vi "运维调试_五参数.vi"() -> ()   [LabVIEW 2016, in "斯坦道多参数.lvlib"]
uses:
  <vilib>/Utility/miscctls.llb/LVPointTypeDef.ctl
  <vilib>/Utility/config.llb/NI_LVConfig.lvlib
panel:
  out "串口号":string
  in  "水深写入":bool
  in  "水深读取":bool
  in  "水深校准":dbl caption="水深校准:"
  in  "仪器参数设置":bool
  out "模块版本号":string
  in  "写入":bool
  in  "读取":bool
  in  "B":dbl caption="校准值B:"
  in  "K":dbl caption="校准值K:"
  in  "标样核查":bool
  in  "串口设置":bool
  in  "质控参数设置":bool
  in  "打开串口":bool
  in  "释放串口":bool
  out "多参数横条运行状态":T1(xcontrol)
  in  "数据区":i32(listbox)
  in  "停止测量(单探)":bool
  in  "启动测量(单探)":bool
  in  "控制命令区探头选择":u16(ring)=9 items=["氨氮"=3, "水温"=9, "pH值"=10, "溶解氧"=11, "电导率"=12, "浊度"=13, "叶绿素a"=14, "藻密度"=15, "蓝绿藻"=16, "氧化还原电位"=17, "溶解氧%"=18, "盐度"=19]
  in  "同步时间":bool
  in  "初始化(清洗)":bool
  in  "停止测量(全部)":bool
  in  "启动测量(全部)":bool
  in  "关键参数区读取":bool
  in  "关键参数区":i32(listbox)
  in  "传感器参数读取":bool
  in  "传感器区":i32(listbox)
  in  "返回":bool
  in  "设置":bool
  out "运行状态":string
  in  "停止":bool
  in  "水样测试":bool
  out "集成报警信息":string
  # "控制命令区"
  # "探头校准"
  # "水深校准"
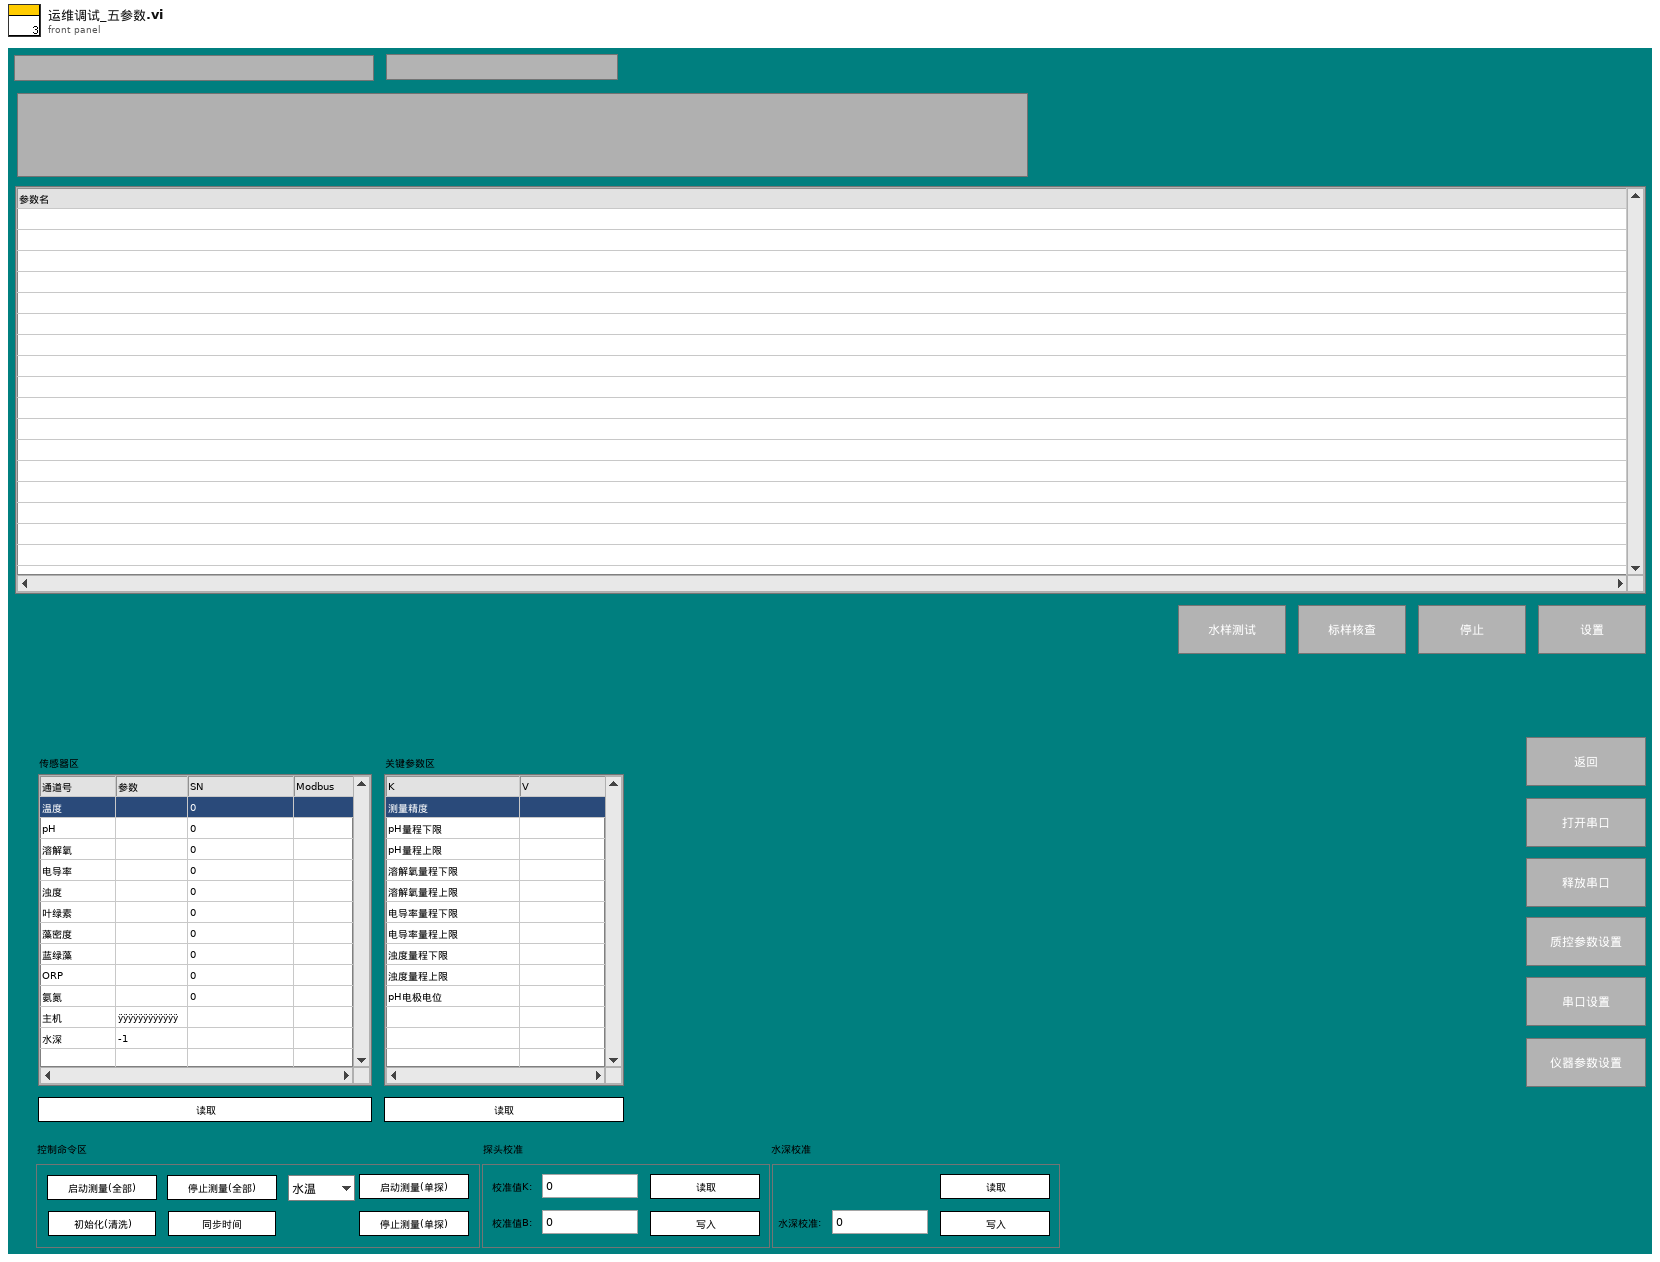
[diagram p1: front panel]
types:
  T1 = cluster{"系统时间":timestamp, "工作状态":u16, "测量模式":u16, "告警代码":enum16{"无告警", "缺试剂告警", "缺水样告警", "缺蒸馏水告警", "缺标液告警", "仪表漏液告警", "标定异常告警", "超量程告警", "加热异常", "低试剂预警", "超上限告警", "超下限告警", "仪表内部其他异常", "滴定异常告警", "电极异常告警", "量程切换告警", "参数设置告警", "PH电极电位异常", "电导率电极异常", "浊度光度异常", "溶解氧电极异常", "溶解氧光强异常", "温度异常告警", "PH异常告警", "溶解氧异常告警", "电导率异常告警", "浊度异常告警", "叶绿素异常告警", "藻密度异常告警", "蓝绿藻异常告警", "ORP异常告警", "氨氮异常告警", "清洁刷异常告警", "SD卡异常告警", "蓝牙异常告警", "Wifi异常告警", "流程异常告警"}, "故障代码":enum16{"无故障", "电机故障", "温度故障", "通讯故障", "滴定故障"}, "日志代码":u16, "软件版本":string}
  T2 = typedef "斯坦道多参数.lvlib/水样测试启动自定义输入参数.ctl" = cluster{"测量模式":enum16{"待机", "水样测试", "标样核查", "零点核查", "跨度核查", "空白测试", "平行样测试", "加标回收", "空白校准", "标样校准", "初始化（清洗）"}, "数据类型":string, "手动启动标记":bool, "测量时间":dbl}
  T3 = typedef "LVPointTypeDef.ctl" = cluster{"Horizontal":i16, "Vertical":i16}
  T4 = cluster{"时间标识":timestamp, "设备":string, "日志信息":string}
  T5 = enum16{"无告警", "缺试剂告警", "缺水样告警", "缺蒸馏水告警", "缺标液告警", "仪表漏液告警", "标定异常告警", "超量程告警", "加热异常", "低试剂预警", "超上限告警", "超下限告警", "仪表内部其他异常", "滴定异常告警", "电极异常告警", "量程切换告警", "参数设置告警", "PH电极电位异常", "电导率电极异常", "浊度光度异常", "溶解氧电极异常", "溶解氧光强异常", "温度异常告警", "PH异常告警", "溶解氧异常告警", "电导率异常告警", "浊度异常告警", "叶绿素异常告警", "藻密度异常告警", "蓝绿藻异常告警", "ORP异常告警", "氨氮异常告警", "清洁刷异常告警", "SD卡异常告警", "蓝牙异常告警", "Wifi异常告警", "流程异常告警"}
  T6 = cluster{"水温":dbl, "pH":dbl, "DO":dbl, "Cond":dbl, "Turb":dbl, "叶绿素":dbl, "藻密度":dbl, "蓝绿藻":dbl, "ORP":dbl, "NH3N":dbl}
  T7 = cluster{"因子编码":string, "单位":string, "标样参考值":sgl, "水样数据时间":timestamp, "水样实测值":sgl, "水样数据标识":string, "K":sgl, "B":sgl, "T":sgl, "H":sgl, "水深":sgl, "探头温度":sgl}
  T8 = typedef "NI_LVConfig.lvlib/Config Data RefNum.ctl" = refnum<k1>
  T9 = cluster{"测量量程":dbl, "测量精度":dbl, "测量间隔":dbl, "消解温度":dbl, "消解时长":dbl, "空白校准时间":timestamp, "曲线截距":dbl, "曲线斜率":dbl, "测量检出限":dbl, "测量信号值":dbl, "线性相关系数":dbl, "二次多项式系数":dbl, "标样校准时间":timestamp, "稀释倍数":dbl, "三项式系数":dbl, "空白标定系数":dbl, "量程系数":dbl, "F0/ORPA":dbl, "F1/ORPB":dbl, "F2/ORPK":dbl, "F3":dbl, "F4":dbl, "F5":dbl, "F6":dbl, "F7":dbl, "X0/滴定数":dbl, "量程":dbl}
  T10 = cluster{"测量量程":dbl, "测量精度":dbl, "测量间隔":dbl, "消解温度":dbl, "消解时长":dbl, "空白校准时间":timestamp, "曲线截距":dbl, "曲线斜率":dbl, "测量检出限":dbl, "测量信号值":dbl, "线性相关系数":dbl, "二次多项式系数":dbl, "标样校准时间":timestamp, "稀释倍数":dbl, "三项式系数":dbl, "空白标定系数":dbl, "量程系数":dbl, "F0/ORPA":dbl, "F1/ORPB":dbl, "F2/ORPK":dbl, "F3":dbl, "F4":dbl, "F5":dbl, "F6":dbl, "F7":dbl, "X0/滴定数":dbl, "量程":dbl}[]
  T11 = cluster{"因子编码":string, "单位":string, "标样参考值":sgl, "水样数据时间":timestamp, "水样实测值":sgl, "水样数据标识":string, "K":sgl, "B":sgl, "T":sgl, "H":sgl, "水深":sgl, "探头温度":sgl}[]
  T12 = enum8{"Enabled", "Disabled", "Disabled and Grayed Out"}
  T13 = typedef "斯坦道多参数.lvlib/标样核查启动自定义输入参数.ctl" = cluster{"测量模式":enum16{"待机", "水样测试", "标样核查", "零点核查", "跨度核查", "空白测试", "平行样测试", "加标回收", "空白校准", "标样校准", "初始化（清洗）"}, "数据标记表":string, "输出参数":cluster{"水温":bool, "pH":bool, "DO":bool, "浊度":bool, "电导率":bool, "保存组数":dbl}}
  T14 = cluster{"水温标准液标准浓度":dbl, "酸碱度标准液标准浓度":dbl, "溶解氧标准液标准浓度":dbl, "电导率标准液标准浓度":dbl, "浊度标准液标准浓度":dbl}
  T15 = cluster{"确定":bool, "水温标准液标准浓度":dbl, "酸碱度标准液标准浓度":dbl, "溶解氧标准液标准浓度":dbl, "电导率标准液标准浓度":dbl, "浊度标准液标准浓度":dbl}
  T16 = cluster{"运行模式":enum16{"维护模式", "常规模式", "应急模式", "质控模式"}, "24H周期设置":bool[]}
  T17 = cluster{"水温":bool, "pH":bool, "DO":bool, "浊度":bool, "电导率":bool, "保存组数":dbl}
  T18 = enum32{"Bad", "Idle", "Run top level", "Running"}
  T19 = cluster{"Major":u16, "Minor":u16, "Fix":u16, "Build":u16}
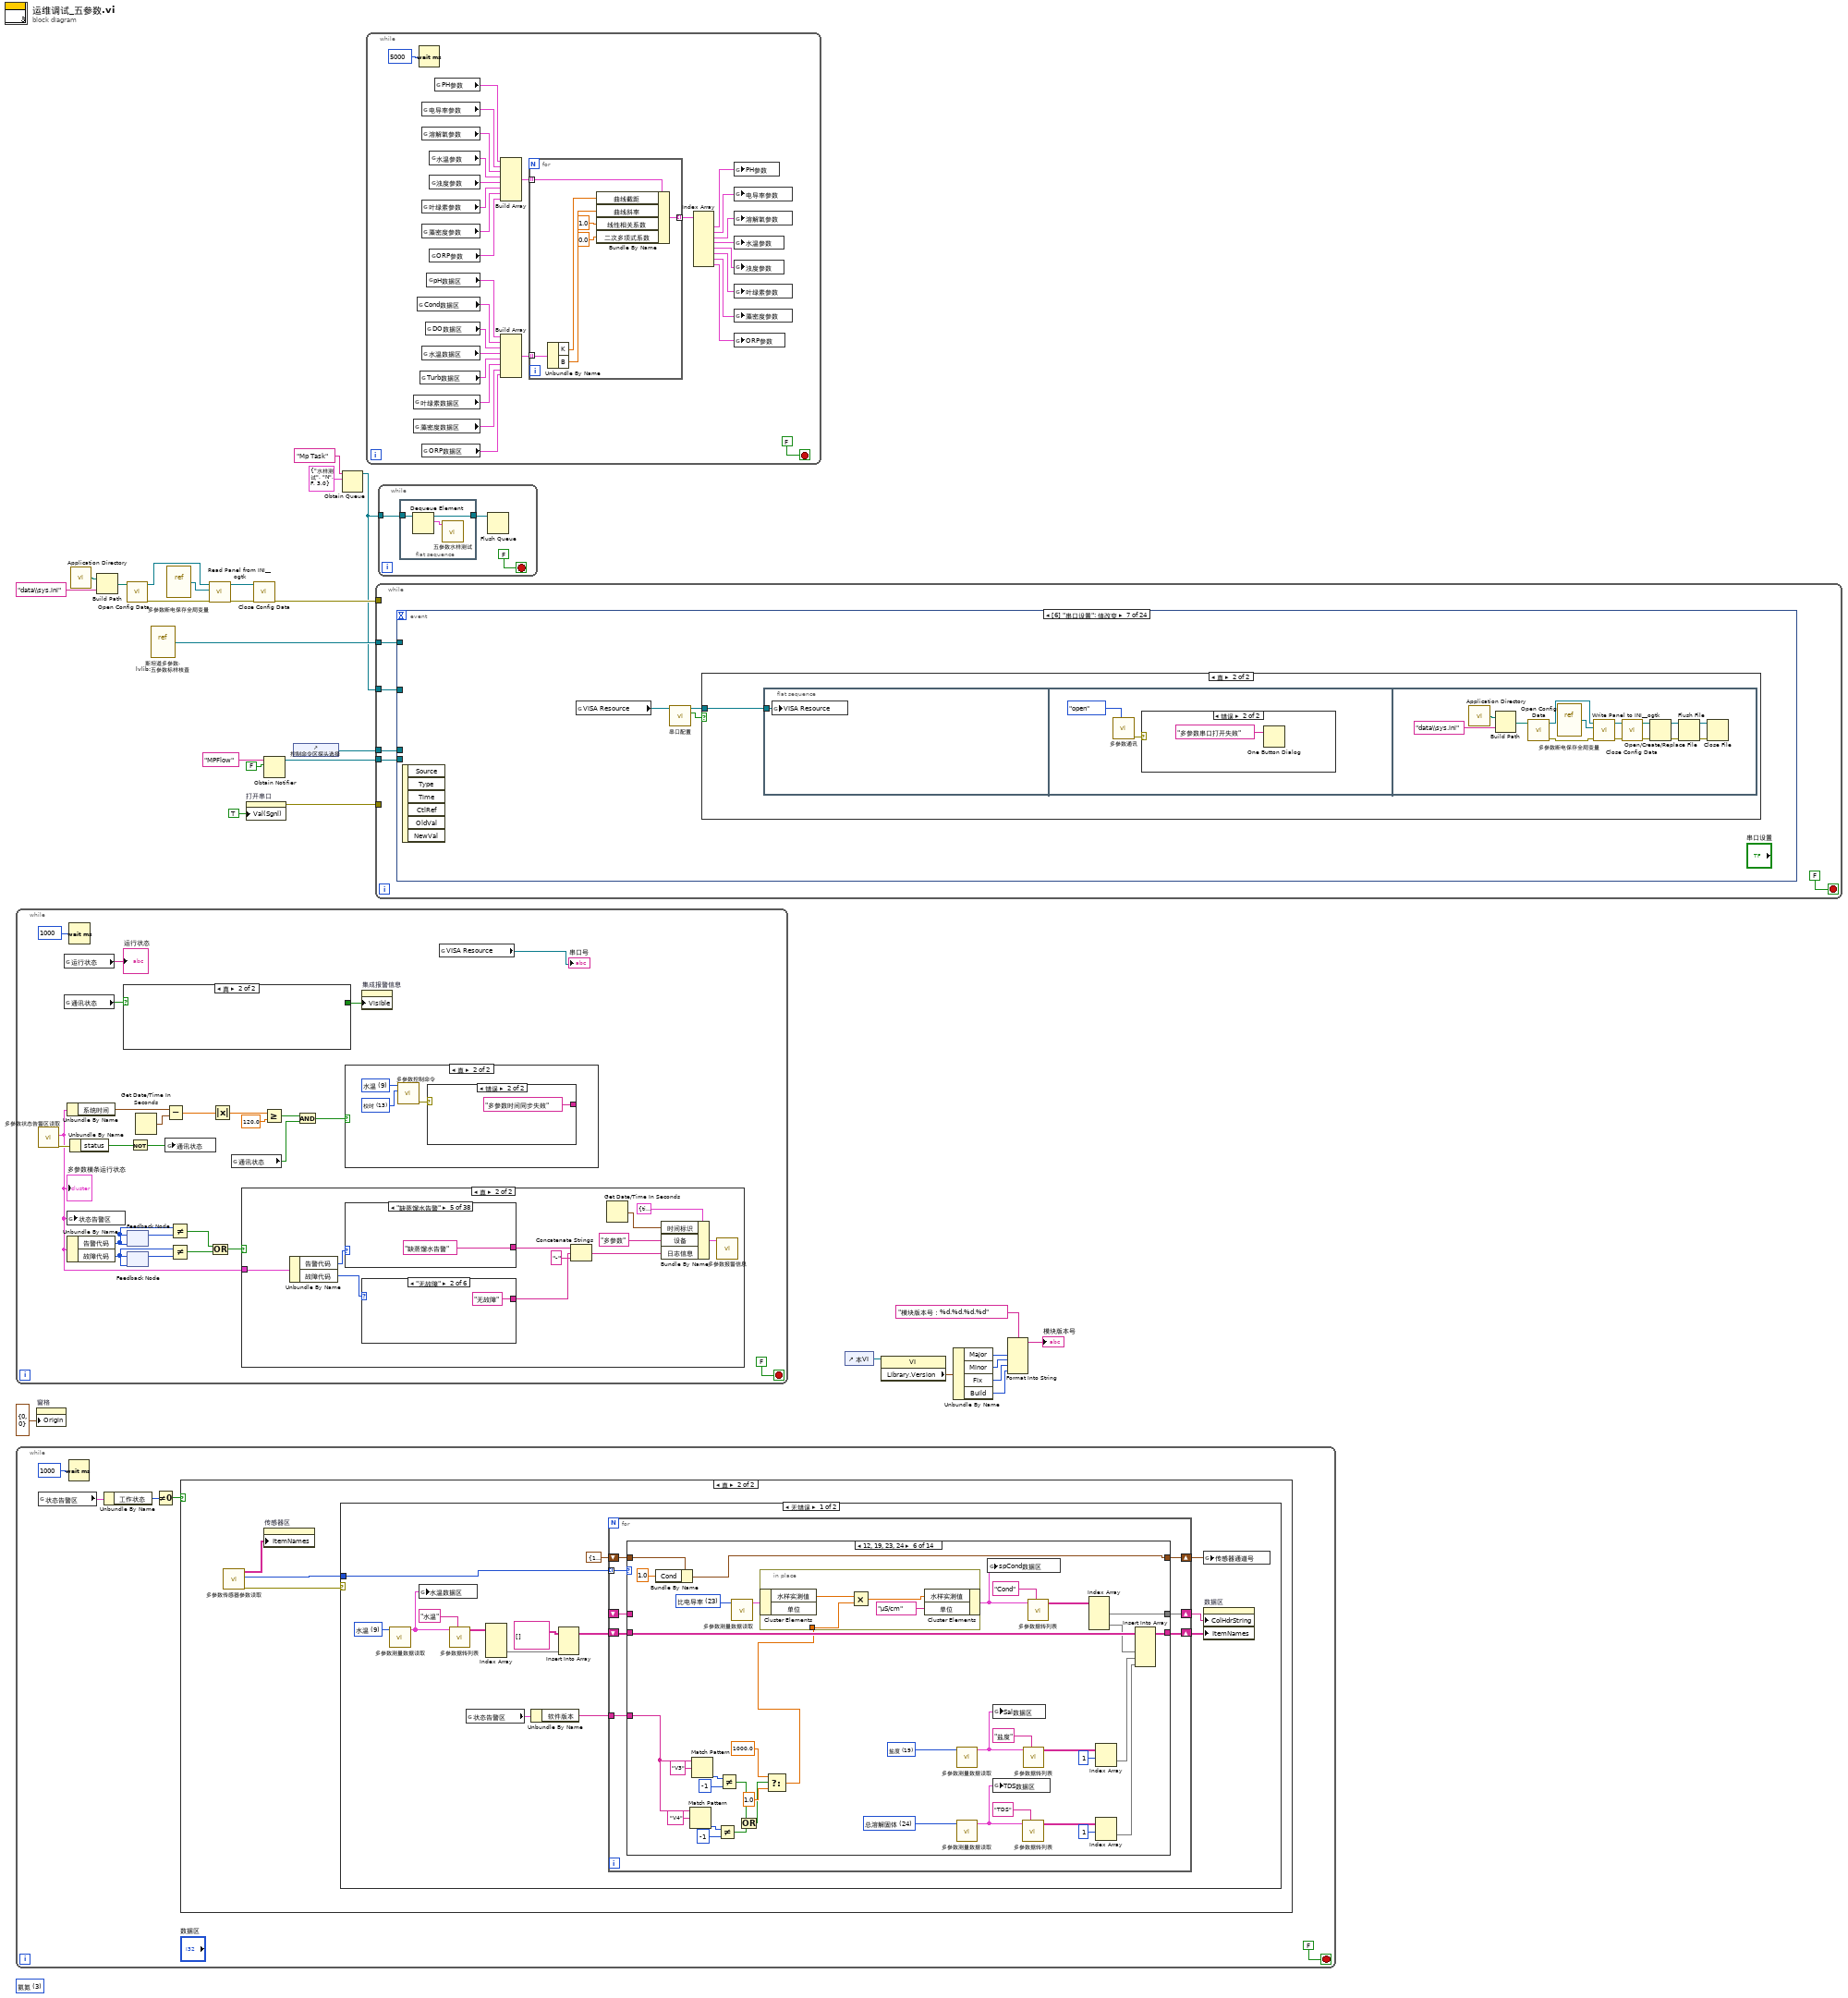
[diagram p0: block diagram]
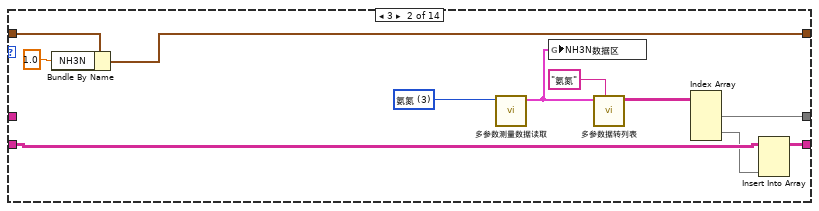
[diagram p4: hidden frame]
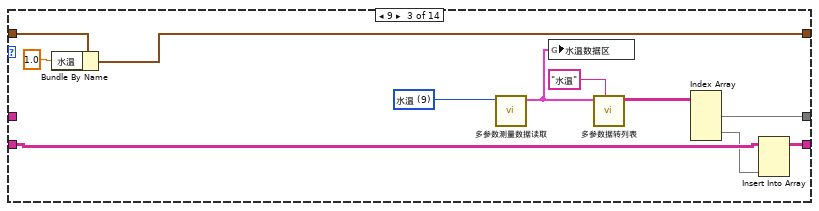
[diagram p5: hidden frame]
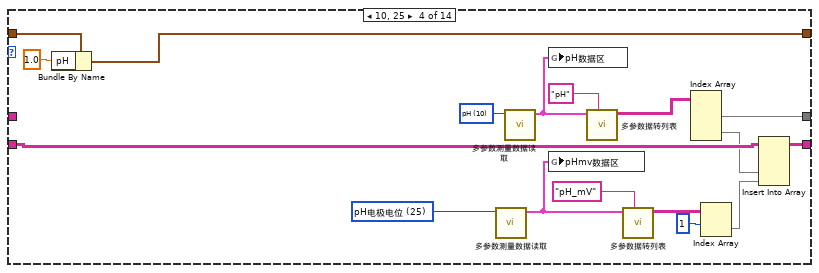
[diagram p6: hidden frame]
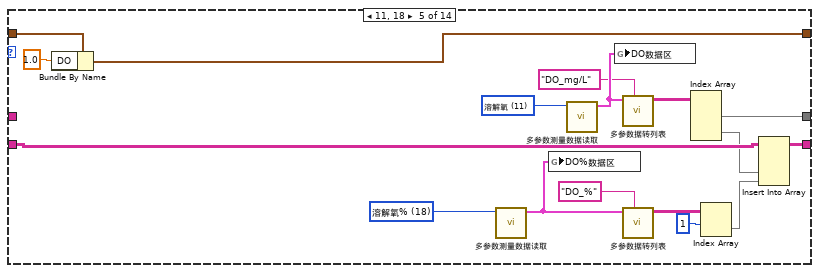
[diagram p7: hidden frame]
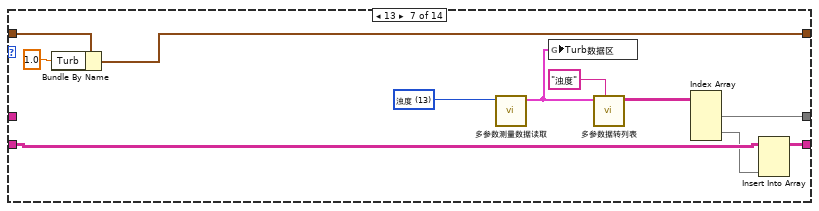
[diagram p8: hidden frame]
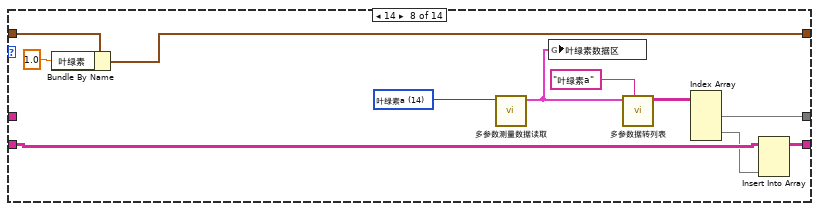
[diagram p9: hidden frame]
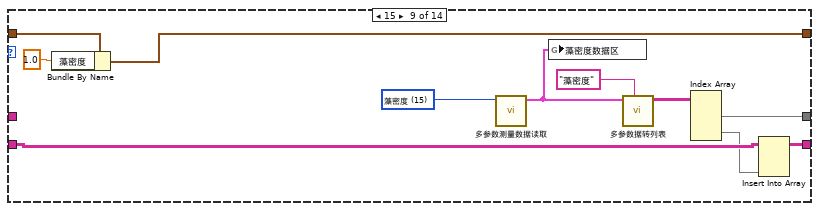
[diagram p10: hidden frame]
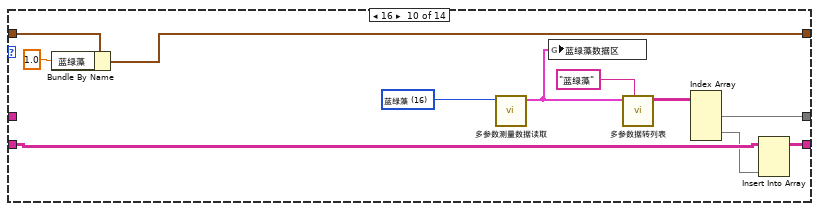
[diagram p11: hidden frame]
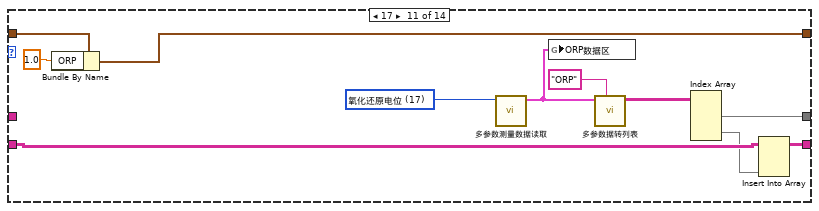
[diagram p12: hidden frame]
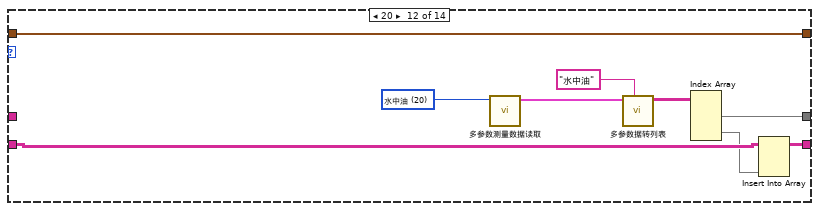
[diagram p13: hidden frame]
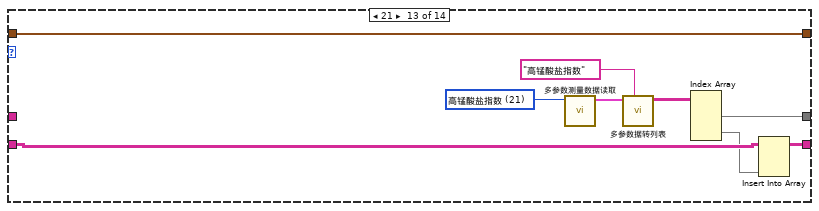
[diagram p14: hidden frame]
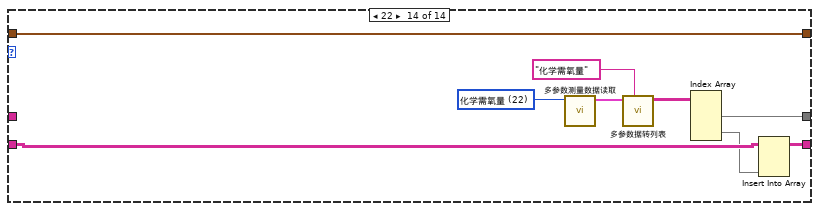
[diagram p15: hidden frame]
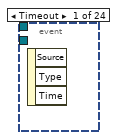
[diagram p17: hidden frame]
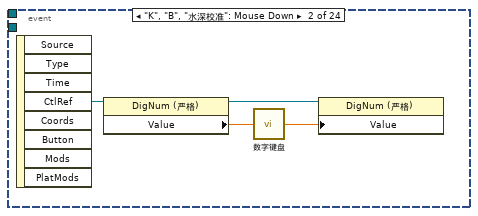
[diagram p18: hidden frame]
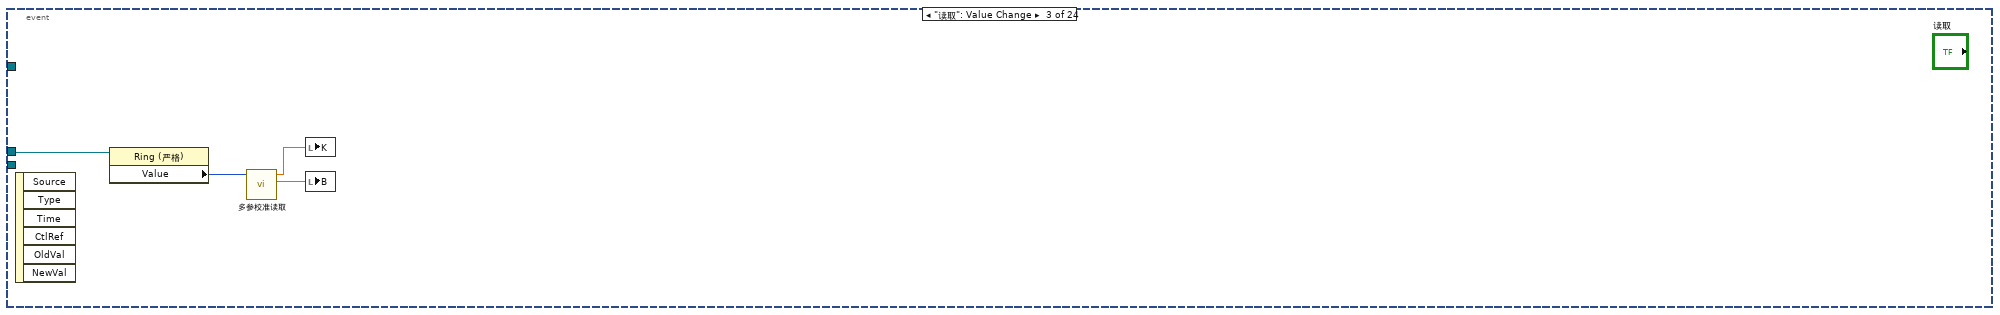
[diagram p19: hidden frame]
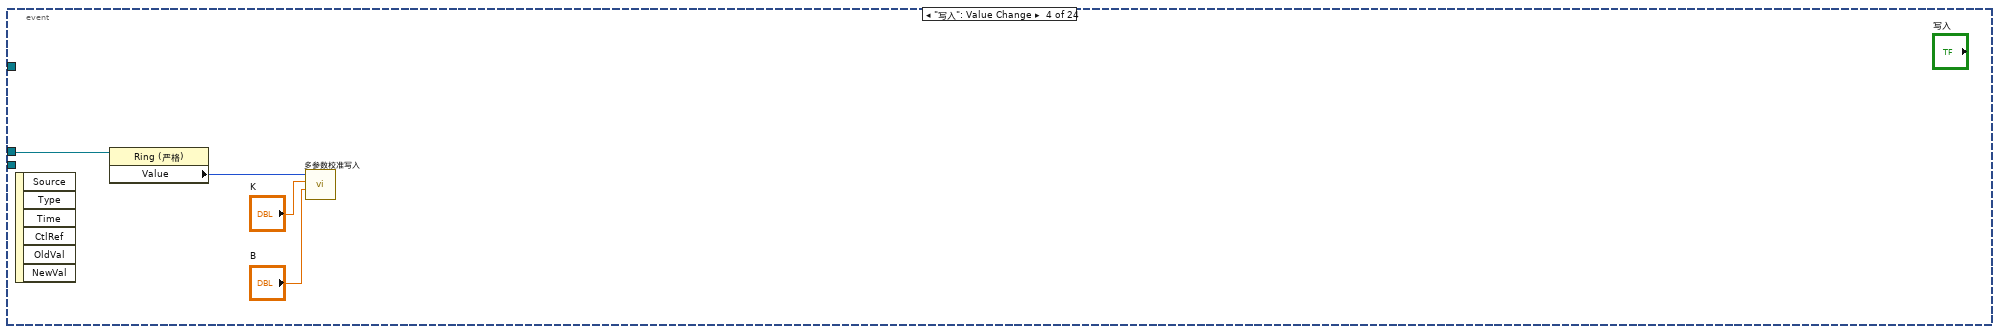
[diagram p20: hidden frame]
diagram:
  (unwired) u16 3 items=["氨氮"=3, "水温"=9, "pH"=10, "溶解氧"=11, "电导率"=12, "浊度"=13, "叶绿素a"=14, "藻密度"=15, "蓝绿藻"=16, "氧化还原电位"=17, "溶解氧%"=18, "盐度"=19, "水中油"=20, "高锰酸盐指数"=21, "化学需氧量"=22, "比电导率"=23, "总溶解固体"=24, "pH电极电位"=25] ("下拉列表")
  n1 = while {
    stop <- FALSE stop-if-true
    n2 = call "多参数状态告警区读取.vi"() -> ("error out"=w41:errorcluster, "状态告警块"=w38:T1)  [unwired: 9 in, 1 out]
    "多参数横条运行状态" <- w38
    n3 = global read "多参数全局变量.vi" "运行状态"() -> (→"运行状态":string)
    n4 = global read "多参数全局变量.vi" "通讯状态"() -> (w51:bool)
    n5 = Unbundle By Name(w38) -> ("系统时间"=w37:timestamp)
    n6 = global write "多参数全局变量.vi" "状态告警区"(w38) -> ()
    n7 = Unbundle By Name(w38) -> ("告警代码"=w47:T5, "故障代码"=w45:enum16{"无故障", "电机故障", "温度故障", "通讯故障", "滴定故障"})
    n8 = Wait (ms)(milliseconds to wait=u32 1000 ("等待时间（毫秒）")) -> ()  [unwired: 1 out]
    n9 = Unbundle By Name(w41) -> ("status"=w40:bool)
    n10 = case shown="真" w51 {
      tunnel: [TRUE ("可见") _] -> w50
      frame False {
        "集成报警信息" <- "通讯异常" ("集成报警信息")
      }
      frame True {
      }
    }
    n11 = feedback #1(w47) -> (w48:T5)
    n12 = feedback-in #1(w47) -> ()
    n13 = feedback #2(w45) -> (w46:enum16{"无故障", "电机故障", "温度故障", "通讯故障", "滴定故障"})
    n14 = feedback-in #2(w45) -> ()
    n15 = Not(x=w40) -> (.not. x?=w39:bool)
    n16 = Get Date/Time In Seconds() -> (seconds since 1Jan1904=w36:timestamp)
    n17 = Subtract(x=w37, y=w36) -> (x-y=w35:dbl)
    n18 = global write "多参数全局变量.vi" "通讯状态"(w39) -> ()
    n19 = Not Equal?(x=w47, y=w48) -> (x != y?=w43:bool)
    n20 = Not Equal?(x=w45, y=w46) -> (x != y?=w44:bool)
    n21 = Or(x=w43, y=w44) -> (x .or. y?=w42:bool)
    n22 = Absolute Value(x=w35) -> (abs(x)=w34:dbl)
    n23 = global read "多参数全局变量.vi" "通讯状态"() -> (w30:bool)
    n24 = case shown="真" w42 {
      tunnel: w38 -> [_ w69]
      frame False {
      }
      frame True {
        n25 = Unbundle By Name(w69) -> ("告警代码"=w68:T5, "故障代码"=w67:enum16{"无故障", "电机故障", "温度故障", "通讯故障", "滴定故障"})
        n26 = case shown="\"缺蒸馏水告警\"" w68 {
          selector: w68 -> [w80 _ _ _ _ _ _ _ _ _ _ _ _ _ _ _ _ _ _ _ _ _ _ _ _ _ _ _ _ _ _ _ _ _ _ _ _ _]
          tunnel: [w79 "无告警" "缺试剂告警" "缺水样告警" "缺蒸馏水告警" "缺标液告警" "仪表漏液告警" "标定异常告警" "超量程告警" "加热异常" "低试剂预警" "超上限告警" "超下限告警" "仪表内部其他异常" "滴定异常告警" "电极异常告警" "量程切换告警" "参数设置告警" "PH电极电位异常" "电导率电极异常" "浊度光度异常" "溶解氧电极异常" "溶解氧光强异常" "温度异常告警" "PH异常告警" "溶解氧异常告警" "电导率异常告警" "浊度异常告警" "叶绿素异常告警" "藻密度异常告警" "蓝绿藻异常告警" "ORP异常告警" "氨氮异常告警" "清洁刷异常告警" "SD卡异常告警" "蓝牙异常告警" "WiFi异常告警" "流程异常告警"] -> w66
          frame Default {
            n27 = Format Into String(format string="%d" ("格式字符串"), initial string="未知" ("工作状态"), w80) -> (resulting string=w79:string)  [unwired: 1 in, 1 out]
          }
          frame "无告警" {
          }
          frame "缺试剂告警" {
          }
          frame "缺水样告警" {
          }
          frame "缺蒸馏水告警" {
          }
          frame "缺标液告警" {
          }
          frame "仪表漏液告警" {
          }
          frame "标定异常告警" {
          }
          frame "超量程告警" {
          }
          frame "加热异常" {
          }
          frame "低试剂预警" {
          }
          frame "超上限告警" {
          }
          frame "超下限告警" {
          }
          frame "仪表内部其他异常" {
          }
          frame "滴定异常告警" {
          }
          frame "电极异常告警" {
          }
          frame "量程切换告警" {
          }
          frame "参数设置告警" {
          }
          frame "PH电极电位异常" {
          }
          frame "电导率电极异常" {
          }
          frame "浊度光度异常" {
          }
          frame "溶解氧电极异常" {
          }
          frame "溶解氧光强异常" {
          }
          frame "温度异常告警" {
          }
          frame "PH异常告警" {
          }
          frame "溶解氧异常告警" {
          }
          frame "电导率异常告警" {
          }
          frame "浊度异常告警" {
          }
          frame "叶绿素异常告警" {
          }
          frame "藻密度异常告警" {
          }
          frame "蓝绿藻异常告警" {
          }
          frame "ORP异常告警" {
          }
          frame "氨氮异常告警" {
          }
          frame "清洁刷异常告警" {
          }
          frame "SD卡异常告警" {
          }
          frame "蓝牙异常告警" {
          }
          frame "Wifi异常告警" {
          }
          frame "流程异常告警" {
          }
        }
        n28 = case shown="\"无故障\"" w67 {
          selector: w67 -> [w71 _ _ _ _ _]
          tunnel: [w70 "无故障" "电机故障" "温度故障" "通讯故障" "滴定故障"] -> w65
          frame Default {
            n29 = Format Into String(format string="%d" ("格式字符串"), initial string="未知" ("工作状态"), w71) -> (resulting string=w70:string)  [unwired: 1 in, 1 out]
          }
          frame "无故障" {
          }
          frame "电机故障" {
          }
          frame "温度故障" {
          }
          frame "通讯故障" {
          }
          frame "滴定故障" {
          }
        }
        n30 = Concatenate Strings(w66, "-" ("字符串"), w65) -> (w61:string)
        n31 = Get Date/Time In Seconds() -> (seconds since 1Jan1904=w60:timestamp)
        n32 = Bundle By Name(cluster=T4 {"时间标识"=timestamp(0 s since 1904-01-01), "设备"="", "日志信息"=""} ("data in"), "时间标识"=w60, "设备"="多参数", "日志信息"=w61) -> (w62:T4)
        n33 = call "多参数报警信息.vi"("data in"=w62) -> ()  [unwired: 10 in, 1 out]
      }
    }
    n34 = Greater Or Equal?(x=w34, y=120.0) -> (x >= y?=w33:bool)
    n35 = And(x=w33, y=w30) -> (x .and. y?=w31:bool)
    n36 = case shown="真" w31 {
      frame False {
      }
      frame True {
        w54 = u16 13 items=["启动测量（全部）"=1, "初始化（清洗）"=10, "停止测量（全部）"=11, "校时"=13, "启动测量（单个传感器）"=19, "停止测量（单个传感器）"=20] ("控制命令")
        w55 = u16 9 items=["氨氮"=3, "水温"=9, "pH值"=10, "溶解氧"=11, "电导率"=12, "浊度"=13, "叶绿素a"=14, "藻密度"=15, "蓝绿藻"=16, "氧化还原电位"=17, "溶解氧%"=18, "盐度"=19] ("站号")
        n37 = call "多参数控制命令.vi"("控制命令"=w54, "站号"=w55) -> ("error out"=w56:errorcluster)  [unwired: 9 in]
        n38 = case shown="错误" w56 {
          tunnel: ["多参数时间同步成功" ("消息") "多参数时间同步失败" ("消息")] -> _
          frame No Error {
          }
          frame Error {
          }
        }
      }
    }
    n39 = property on="集成报警信息" class="Str"("Visible"=w50) -> ()  [unwired: 2 in, 2 out]
    n40 = global read "多参数断电保存全局变量.vi" "VISA Resource"() -> (→"串口号":refnum<visa-resource-name>)
  }
  n41 = while {
    stop <- FALSE stop-if-true
    n42 = global read "多参数全局变量.vi" "状态告警区"() -> (w124:T1)
    n43 = Wait (ms)(milliseconds to wait=u32 1000 ("等待时间（毫秒）")) -> ()  [unwired: 1 out]
    n44 = Unbundle By Name(w124) -> ("工作状态"=w123:u16)
    n45 = Not Equal To 0?(x=w123) -> (x != 0?=w122:bool)
    n46 = case shown="真" w122 {
      frame False {
      }
      frame True {
        n47 = call "多参数传感器参数读取.vi"() -> ("error out"=w129:errorcluster, "modbus"=w128:u16[], "添加的数组"=w127:string[][])  [unwired: 9 in]
        n48 = property on="传感器区" class="MCListbox (严格)"("ItemNames"=w127) -> ()  [unwired: 2 in, 2 out]
        n49 = case shown="无错误" w129 {
          tunnel: w128 -> [w143 _]
          frame No Error {
            w140 = u16 9 items=["氨氮"=3, "水温"=9, "pH"=10, "溶解氧"=11, "电导率"=12, "浊度"=13, "叶绿素a"=14, "藻密度"=15, "蓝绿藻"=16, "氧化还原电位"=17, "溶解氧%"=18, "盐度"=19, "水中油"=20, "高锰酸盐指数"=21, "化学需氧量"=22, "比电导率"=23, "总溶解固体"=24, "pH电极电位"=25] ("下拉列表")
            n50 = call "多参数测量数据读取.vi"("探头选择"=w140) -> ("测量数据块"=w135:T7)  [unwired: 8 in, 2 out]
            n51 = global write "多参数全局变量.vi" "水温数据区"(w135) -> ()
            n52 = call "多参数据转列表.vi"("参数名"="水温", "测量数据块"=w135) -> ("添加的数组"=w133:string[][])  [unwired: 9 in]
            n53 = global read "多参数全局变量.vi" "状态告警区"() -> (w131:T1)
            n54 = Index Array(array=w133) -> (element #2=w132:string[])  [unwired: 4 in, 1 out]
            n55 = Unbundle By Name(w131) -> ("软件版本"=w130:string)
            n56 = Insert Into Array(array=string[][] [] ("子数组"), new element=w132) -> (w138:string[][])  [unwired: 2 in]
            n57 = for {
              tunnel: w143 -> [w151] mode=indexing
              shift-right: [w149] -> w141
              shift-left: w138 -> [w150]
              shift-right: [w148] -> w142
              shift-left: _ -> [w147]
              shift-right: [w146] -> w136
              shift-left: T6 {"水温"=1.0, "pH"=0.0, "DO"=0.0, "Cond"=0.0, "Turb"=0.0, "叶绿素"=0.0, "藻密度"=0.0, "蓝绿藻"=0.0, "ORP"=0.0, "NH3N"=0.0} ("传感器通道号") -> [w145]
              tunnel: w130 -> [w144]
              n58 = case shown="12, 19, 23, 24" w151 {
                tunnel: w150 -> [w154 w164 w175 w192 w209 w246 w261 w272 w283 w294 w305 w314 w323 w332]
                tunnel: [w154 w163 w174 w191 w208 w245 w260 w271 w282 w293 w304 w313 w322 w331] -> w149
                tunnel: [w153 w156 w167 w184 w201 w237 w254 w264 w277 w287 w298 w308 w317 w326] -> w148
                tunnel: w147 -> [w153 _ _ _ _ _ _ _ _ _ _ _ _ _]
                tunnel: [w152 w160 w171 w187 w205 w240 w257 w268 w279 w290 w301 w312 w321 w330] -> w146
                tunnel: w145 -> [w152 w162 w173 w189 w207 w241 w258 w269 w280 w291 w302 w312 w321 w330]
                tunnel: w144 -> [_ _ _ _ _ w216 _ _ _ _ _ _ _ _]
                frame 0, Default {
                }
                frame 3 {
                  w165 = u16 3 items=["氨氮"=3, "水温"=9, "pH"=10, "溶解氧"=11, "电导率"=12, "浊度"=13, "叶绿素a"=14, "藻密度"=15, "蓝绿藻"=16, "氧化还原电位"=17, "溶解氧%"=18, "盐度"=19, "水中油"=20, "高锰酸盐指数"=21, "化学需氧量"=22, "比电导率"=23, "总溶解固体"=24, "pH电极电位"=25] ("下拉列表")
                  n59 = Bundle By Name(cluster=w162, "NH3N"=1.0) -> (w160:T6)
                  n60 = call "多参数测量数据读取.vi"("探头选择"=w165) -> ("测量数据块"=w159:T7)  [unwired: 8 in, 2 out]
                  n61 = global write "多参数全局变量.vi" "NH3N数据区"(w159) -> ()
                  n62 = call "多参数据转列表.vi"("参数名"="氨氮", "测量数据块"=w159) -> ("添加的数组"=w158:string[][])  [unwired: 9 in]
                  n63 = Index Array(array=w158) -> (element #1=w156:string[], element #2=w155:string[])  [unwired: 4 in]
                  n64 = Insert Into Array(array=w164, new element=w155) -> (w163:string[][])  [unwired: 2 in]
                }
                frame 9 {
                  w176 = u16 9 items=["氨氮"=3, "水温"=9, "pH"=10, "溶解氧"=11, "电导率"=12, "浊度"=13, "叶绿素a"=14, "藻密度"=15, "蓝绿藻"=16, "氧化还原电位"=17, "溶解氧%"=18, "盐度"=19, "水中油"=20, "高锰酸盐指数"=21, "化学需氧量"=22, "比电导率"=23, "总溶解固体"=24, "pH电极电位"=25] ("下拉列表")
                  n65 = Bundle By Name(cluster=w173, "水温"=1.0) -> (w171:T6)
                  n66 = call "多参数测量数据读取.vi"("探头选择"=w176) -> ("测量数据块"=w170:T7)  [unwired: 8 in, 2 out]
                  n67 = global write "多参数全局变量.vi" "水温数据区"(w170) -> ()
                  n68 = call "多参数据转列表.vi"("参数名"="水温", "测量数据块"=w170) -> ("添加的数组"=w169:string[][])  [unwired: 9 in]
                  n69 = Index Array(array=w169) -> (element #1=w167:string[], element #2=w166:string[])  [unwired: 4 in]
                  n70 = Insert Into Array(array=w175, new element=w166) -> (w174:string[][])  [unwired: 2 in]
                }
                frame 10, 25 {
                  w190 = u16 25 items=["氨氮"=3, "水温"=9, "pH"=10, "溶解氧"=11, "电导率"=12, "浊度"=13, "叶绿素a"=14, "藻密度"=15, "蓝绿藻"=16, "氧化还原电位"=17, "溶解氧%"=18, "盐度"=19, "水中油"=20, "高锰酸盐指数"=21, "化学需氧量"=22, "比电导率"=23, "总溶解固体"=24, "pH电极电位"=25] ("下拉列表")
                  w193 = u16 10 items=["氨氮"=3, "水温"=9, "pH"=10, "溶解氧"=11, "电导率"=12, "浊度"=13, "叶绿素a"=14, "藻密度"=15, "蓝绿藻"=16, "氧化还原电位"=17, "溶解氧%"=18, "盐度"=19, "水中油"=20, "高锰酸盐指数"=21, "化学需氧量"=22, "比电导率"=23, "总溶解固体"=24, "pH电极电位"=25] ("下拉列表")
                  n71 = Bundle By Name(cluster=w189, "pH"=1.0) -> (w187:T6)
                  n72 = call "多参数测量数据读取.vi"("探头选择"=w190) -> ("测量数据块"=w180:T7)  [unwired: 8 in, 2 out]
                  n73 = call "多参数测量数据读取.vi"("探头选择"=w193) -> ("测量数据块"=w186:T7)  [unwired: 8 in, 2 out]
                  n74 = global write "多参数全局变量.vi" "pH数据区"(w186) -> ()
                  n75 = global write "多参数全局变量.vi" "pHmv数据区"(w180) -> ()
                  n76 = call "多参数据转列表.vi"("参数名"="pH", "测量数据块"=w186) -> ("添加的数组"=w185:string[][])  [unwired: 9 in]
                  n77 = call "多参数据转列表.vi"("参数名"="pH_mV", "测量数据块"=w180) -> ("添加的数组"=w179:string[][])  [unwired: 9 in]
                  n78 = Index Array(array=w185) -> (element #1=w184:string[], element #2=w183:string[])  [unwired: 4 in]
                  n79 = Index Array(array=w179, index (row)=1 ("禁用的索引 (列)")) -> (element=w182:string[])  [unwired: 1 in]
                  n80 = Insert Into Array(array=w192, new element #1=w183, new element #2=w182) -> (w191:string[][])  [unwired: 2 in]
                }
                frame 11, 18 {
                  w199 = u16 18 items=["氨氮"=3, "水温"=9, "pH"=10, "溶解氧"=11, "电导率"=12, "浊度"=13, "叶绿素a"=14, "藻密度"=15, "蓝绿藻"=16, "氧化还原电位"=17, "溶解氧%"=18, "盐度"=19, "水中油"=20, "高锰酸盐指数"=21, "化学需氧量"=22, "比电导率"=23, "总溶解固体"=24, "pH电极电位"=25] ("下拉列表")
                  w210 = u16 11 items=["氨氮"=3, "水温"=9, "pH"=10, "溶解氧"=11, "电导率"=12, "浊度"=13, "叶绿素a"=14, "藻密度"=15, "蓝绿藻"=16, "氧化还原电位"=17, "溶解氧%"=18, "盐度"=19, "水中油"=20, "高锰酸盐指数"=21, "化学需氧量"=22, "比电导率"=23, "总溶解固体"=24, "pH电极电位"=25] ("下拉列表")
                  n81 = Bundle By Name(cluster=w207, "DO"=1.0) -> (w205:T6)
                  n82 = call "多参数测量数据读取.vi"("探头选择"=w199) -> ("测量数据块"=w198:T7)  [unwired: 8 in, 2 out]
                  n83 = global write "多参数全局变量.vi" "DO%数据区"(w198) -> ()
                  n84 = call "多参数测量数据读取.vi"("探头选择"=w210) -> ("测量数据块"=w204:T7)  [unwired: 8 in, 2 out]
                  n85 = global write "多参数全局变量.vi" "DO数据区"(w204) -> ()
                  n86 = call "多参数据转列表.vi"("参数名"="DO_mg/L", "测量数据块"=w204) -> ("添加的数组"=w202:string[][])  [unwired: 9 in]
                  n87 = call "多参数据转列表.vi"("参数名"="DO_%", "测量数据块"=w198) -> ("添加的数组"=w196:string[][])  [unwired: 9 in]
                  n88 = Index Array(array=w202) -> (element #1=w201:string[], element #2=w200:string[])  [unwired: 4 in]
                  n89 = Index Array(array=w196, index (row)=1 ("禁用的索引 (列)")) -> (element=w195:string[])  [unwired: 1 in]
                  n90 = Insert Into Array(array=w209, new element #1=w200, new element #2=w195) -> (w208:string[][])  [unwired: 2 in]
                }
                frame 12, 19, 23, 24 {
                  w243 = u16 24 items=["氨氮"=3, "水温"=9, "pH"=10, "溶解氧"=11, "电导率"=12, "浊度"=13, "叶绿素a"=14, "藻密度"=15, "蓝绿藻"=16, "氧化还原电位"=17, "溶解氧%"=18, "盐度"=19, "水中油"=20, "高锰酸盐指数"=21, "化学需氧量"=22, "比电导率"=23, "总溶解固体"=24, "pH电极电位"=25] ("下拉列表")
                  w244 = u16 19 items=["氨氮"=3, "水温"=9, "pH"=10, "溶解氧"=11, "电导率"=12, "浊度"=13, "叶绿素a"=14, "藻密度"=15, "蓝绿藻"=16, "氧化还原电位"=17, "溶解氧%"=18, "盐度"=19, "水中油"=20, "高锰酸盐指数"=21, "化学需氧量"=22, "比电导率"=23, "总溶解固体"=24, "pH电极电位"=25] ("下拉列表")
                  w247 = u16 23 items=["氨氮"=3, "水温"=9, "pH"=10, "溶解氧"=11, "电导率"=12, "浊度"=13, "叶绿素a"=14, "藻密度"=15, "蓝绿藻"=16, "氧化还原电位"=17, "溶解氧%"=18, "盐度"=19, "水中油"=20, "高锰酸盐指数"=21, "化学需氧量"=22, "比电导率"=23, "总溶解固体"=24, "pH电极电位"=25] ("下拉列表")
                  n91 = Bundle By Name(cluster=w241, "Cond"=1.0 ("DO")) -> (w240:T6)
                  n92 = Match Pattern(string=w216, regular expression="V4" ("正则表达式")) -> (offset past match=w218:i32)  [unwired: 1 in, 3 out]
                  n93 = Match Pattern(string=w216, regular expression="V3" ("正则表达式")) -> (offset past match=w224:i32)  [unwired: 1 in, 3 out]
                  n94 = Not Equal?(x=w218, y=-1) -> (x != y?=w215:bool)
                  n95 = Not Equal?(x=w224, y=-1) -> (x != y?=w214:bool)
                  n96 = call "多参数测量数据读取.vi"("探头选择"=w247) -> ("测量数据块"=w229:T7)  [unwired: 8 in, 2 out]
                  n97 = Or(x=w214, y=w215) -> (x .or. y?=w213:bool)
                  n98 = Select(t=1000.0, s=w213, f=1.0) -> (s? t:f=w220:dbl)
                  n99 = in-place {
                    in-place-border: w220 -> [w248]
                    n100 = in-place-cluster #3(w229) -> ("水样实测值"=w250:sgl)  [unwired: 1 out]
                    n101 = Multiply(x=w250, y=w248) -> (x*y=w249:dbl)
                    n102 = in-place-cluster #3("水样实测值"=w249, "单位"="μS/cm") -> (w228:T7)
                  }
                  n103 = call "多参数测量数据读取.vi"("探头选择"=w244) -> ("测量数据块"=w234:T7)  [unwired: 8 in, 2 out]
                  n104 = call "多参数测量数据读取.vi"("探头选择"=w243) -> ("测量数据块"=w231:T7)  [unwired: 8 in, 2 out]
                  n105 = global write "多参数全局变量.vi" "spCond数据区"(w228) -> ()
                  n106 = global write "多参数全局变量.vi" "Sal数据区"(w234) -> ()
                  n107 = global write "多参数全局变量.vi" "TDS数据区"(w231) -> ()
                  n108 = call "多参数据转列表.vi"("参数名"="TDS", "测量数据块"=w231) -> ("添加的数组"=w230:string[][])  [unwired: 9 in]
                  n109 = call "多参数据转列表.vi"("参数名"="盐度", "测量数据块"=w234) -> ("添加的数组"=w233:string[][])  [unwired: 9 in]
                  n110 = call "多参数据转列表.vi"("参数名"="Cond", "测量数据块"=w228) -> ("添加的数组"=w238:string[][])  [unwired: 9 in]
                  n111 = Index Array(array=w238) -> (element #1=w237:string[], element #2=w236:string[])  [unwired: 4 in]
                  n112 = Index Array(array=w233, index (row)=1 ("禁用的索引 (列)")) -> (element=w212:string[])  [unwired: 1 in]
                  n113 = Index Array(array=w230, index (row)=1 ("禁用的索引 (列)")) -> (element=w211:string[])  [unwired: 1 in]
                  n114 = Insert Into Array(array=w246, new element #1=w236, new element #2=w212, new element #3=w211) -> (w245:string[][])  [unwired: 2 in]
                }
                frame 13 {
                  w262 = u16 13 items=["氨氮"=3, "水温"=9, "pH"=10, "溶解氧"=11, "电导率"=12, "浊度"=13, "叶绿素a"=14, "藻密度"=15, "蓝绿藻"=16, "氧化还原电位"=17, "溶解氧%"=18, "盐度"=19, "水中油"=20, "高锰酸盐指数"=21, "化学需氧量"=22, "比电导率"=23, "总溶解固体"=24, "pH电极电位"=25] ("下拉列表")
                  n115 = Bundle By Name(cluster=w258, "Turb"=1.0 ("DO")) -> (w257:T6)
                  n116 = call "多参数测量数据读取.vi"("探头选择"=w262) -> ("测量数据块"=w252:T7)  [unwired: 8 in, 2 out]
                  n117 = global write "多参数全局变量.vi" "Turb数据区"(w252) -> ()
                  n118 = call "多参数据转列表.vi"("参数名"="浊度", "测量数据块"=w252) -> ("添加的数组"=w255:string[][])  [unwired: 9 in]
                  n119 = Index Array(array=w255) -> (element #1=w254:string[], element #2=w253:string[])  [unwired: 4 in]
                  n120 = Insert Into Array(array=w261, new element=w253) -> (w260:string[][])  [unwired: 2 in]
                }
                frame 14 {
                  w273 = u16 14 items=["氨氮"=3, "水温"=9, "pH"=10, "溶解氧"=11, "电导率"=12, "浊度"=13, "叶绿素a"=14, "藻密度"=15, "蓝绿藻"=16, "氧化还原电位"=17, "溶解氧%"=18, "盐度"=19, "水中油"=20, "高锰酸盐指数"=21, "化学需氧量"=22, "比电导率"=23, "总溶解固体"=24, "pH电极电位"=25] ("下拉列表")
                  n121 = Bundle By Name(cluster=w269, "叶绿素"=1.0 ("DO")) -> (w268:T6)
                  n122 = call "多参数测量数据读取.vi"("探头选择"=w273) -> ("测量数据块"=w267:T7)  [unwired: 8 in, 2 out]
                  n123 = global write "多参数全局变量.vi" "叶绿素数据区"(w267) -> ()
                  n124 = call "多参数据转列表.vi"("参数名"="叶绿素a", "测量数据块"=w267) -> ("添加的数组"=w265:string[][])  [unwired: 9 in]
                  n125 = Index Array(array=w265) -> (element #1=w264:string[], element #2=w263:string[])  [unwired: 4 in]
                  n126 = Insert Into Array(array=w272, new element=w263) -> (w271:string[][])  [unwired: 2 in]
                }
                frame 15 {
                  w284 = u16 15 items=["氨氮"=3, "水温"=9, "pH"=10, "溶解氧"=11, "电导率"=12, "浊度"=13, "叶绿素a"=14, "藻密度"=15, "蓝绿藻"=16, "氧化还原电位"=17, "溶解氧%"=18, "盐度"=19, "水中油"=20, "高锰酸盐指数"=21, "化学需氧量"=22, "比电导率"=23, "总溶解固体"=24, "pH电极电位"=25] ("下拉列表")
                  n127 = Bundle By Name(cluster=w280, "藻密度"=1.0 ("DO")) -> (w279:T6)
                  n128 = call "多参数测量数据读取.vi"("探头选择"=w284) -> ("测量数据块"=w276:T7)  [unwired: 8 in, 2 out]
                  n129 = global write "多参数全局变量.vi" "藻密度数据区"(w276) -> ()
                  n130 = call "多参数据转列表.vi"("参数名"="藻密度", "测量数据块"=w276) -> ("添加的数组"=w278:string[][])  [unwired: 9 in]
                  n131 = Index Array(array=w278) -> (element #1=w277:string[], element #2=w275:string[])  [unwired: 4 in]
                  n132 = Insert Into Array(array=w283, new element=w275) -> (w282:string[][])  [unwired: 2 in]
                }
                frame 16 {
                  w295 = u16 16 items=["氨氮"=3, "水温"=9, "pH"=10, "溶解氧"=11, "电导率"=12, "浊度"=13, "叶绿素a"=14, "藻密度"=15, "蓝绿藻"=16, "氧化还原电位"=17, "溶解氧%"=18, "盐度"=19, "水中油"=20, "高锰酸盐指数"=21, "化学需氧量"=22, "比电导率"=23, "总溶解固体"=24, "pH电极电位"=25] ("下拉列表")
                  n133 = Bundle By Name(cluster=w291, "蓝绿藻"=1.0 ("DO")) -> (w290:T6)
                  n134 = call "多参数测量数据读取.vi"("探头选择"=w295) -> ("测量数据块"=w289:T7)  [unwired: 8 in, 2 out]
                  n135 = global write "多参数全局变量.vi" "蓝绿藻数据区"(w289) -> ()
                  n136 = call "多参数据转列表.vi"("参数名"="蓝绿藻", "测量数据块"=w289) -> ("添加的数组"=w288:string[][])  [unwired: 9 in]
                  n137 = Index Array(array=w288) -> (element #1=w287:string[], element #2=w286:string[])  [unwired: 4 in]
                  n138 = Insert Into Array(array=w294, new element=w286) -> (w293:string[][])  [unwired: 2 in]
                }
                frame 17 {
                  w306 = u16 17 items=["氨氮"=3, "水温"=9, "pH"=10, "溶解氧"=11, "电导率"=12, "浊度"=13, "叶绿素a"=14, "藻密度"=15, "蓝绿藻"=16, "氧化还原电位"=17, "溶解氧%"=18, "盐度"=19, "水中油"=20, "高锰酸盐指数"=21, "化学需氧量"=22, "比电导率"=23, "总溶解固体"=24, "pH电极电位"=25] ("下拉列表")
                  n139 = Bundle By Name(cluster=w302, "ORP"=1.0 ("DO")) -> (w301:T6)
                  n140 = call "多参数测量数据读取.vi"("探头选择"=w306) -> ("测量数据块"=w300:T7)  [unwired: 8 in, 2 out]
                  n141 = global write "多参数全局变量.vi" "ORP数据区"(w300) -> ()
                  n142 = call "多参数据转列表.vi"("参数名"="ORP", "测量数据块"=w300) -> ("添加的数组"=w299:string[][])  [unwired: 9 in]
                  n143 = Index Array(array=w299) -> (element #1=w298:string[], element #2=w296:string[])  [unwired: 4 in]
                  n144 = Insert Into Array(array=w305, new element=w296) -> (w304:string[][])  [unwired: 2 in]
                }
                frame 20 {
                  w315 = u16 20 items=["氨氮"=3, "水温"=9, "pH"=10, "溶解氧"=11, "电导率"=12, "浊度"=13, "叶绿素a"=14, "藻密度"=15, "蓝绿藻"=16, "氧化还原电位"=17, "溶解氧%"=18, "盐度"=19, "水中油"=20, "高锰酸盐指数"=21, "化学需氧量"=22, "比电导率"=23, "总溶解固体"=24, "pH电极电位"=25] ("下拉列表")
                  n145 = call "多参数测量数据读取.vi"("探头选择"=w315) -> ("测量数据块"=w311:T7)  [unwired: 8 in, 2 out]
                  n146 = call "多参数据转列表.vi"("参数名"="水中油", "测量数据块"=w311) -> ("添加的数组"=w309:string[][])  [unwired: 9 in]
                  n147 = Index Array(array=w309) -> (element #1=w308:string[], element #2=w307:string[])  [unwired: 4 in]
                  n148 = Insert Into Array(array=w314, new element=w307) -> (w313:string[][])  [unwired: 2 in]
                }
                frame 21 {
                  w324 = u16 21 items=["氨氮"=3, "水温"=9, "pH"=10, "溶解氧"=11, "电导率"=12, "浊度"=13, "叶绿素a"=14, "藻密度"=15, "蓝绿藻"=16, "氧化还原电位"=17, "溶解氧%"=18, "盐度"=19, "水中油"=20, "高锰酸盐指数"=21, "化学需氧量"=22, "比电导率"=23, "总溶解固体"=24, "pH电极电位"=25] ("下拉列表")
                  n149 = call "多参数测量数据读取.vi"("探头选择"=w324) -> ("测量数据块"=w320:T7)  [unwired: 8 in, 2 out]
                  n150 = call "多参数据转列表.vi"("参数名"="高锰酸盐指数", "测量数据块"=w320) -> ("添加的数组"=w319:string[][])  [unwired: 9 in]
                  n151 = Index Array(array=w319) -> (element #1=w317:string[], element #2=w316:string[])  [unwired: 4 in]
                  n152 = Insert Into Array(array=w323, new element=w316) -> (w322:string[][])  [unwired: 2 in]
                }
                frame 22 {
                  w333 = u16 22 items=["氨氮"=3, "水温"=9, "pH"=10, "溶解氧"=11, "电导率"=12, "浊度"=13, "叶绿素a"=14, "藻密度"=15, "蓝绿藻"=16, "氧化还原电位"=17, "溶解氧%"=18, "盐度"=19, "水中油"=20, "高锰酸盐指数"=21, "化学需氧量"=22, "比电导率"=23, "总溶解固体"=24, "pH电极电位"=25] ("下拉列表")
                  n153 = call "多参数测量数据读取.vi"("探头选择"=w333) -> ("测量数据块"=w329:T7)  [unwired: 8 in, 2 out]
                  n154 = call "多参数据转列表.vi"("参数名"="化学需氧量", "测量数据块"=w329) -> ("添加的数组"=w328:string[][])  [unwired: 9 in]
                  n155 = Index Array(array=w328) -> (element #1=w326:string[], element #2=w325:string[])  [unwired: 4 in]
                  n156 = Insert Into Array(array=w332, new element=w325) -> (w331:string[][])  [unwired: 2 in]
                }
              }
            }
            n157 = global write "多参数全局变量.vi" "传感器通道号"(w136) -> ()
            n158 = property on="数据区" class="MCListbox (严格)"("ColHdrString"=w142, "ItemNames"=w141) -> ()  [unwired: 2 in, 2 out]
          }
          frame Error {
          }
        }
      }
    }
  }
  n159 = property on="窗格" class="Pane"("Origin"=T3 {"Horizontal"=0, "Vertical"=0} ("原点")) -> ()  [unwired: 2 in, 2 out]
  n160 = call <vilib>:"Application Directory.vi"() -> ("Application Directory"=w14:path)
  n161 = Build Path(base path=w14, name or relative path="data\\sys.ini" ("名称或相对路径")) -> (appended path=w16:path)
  n162 = call <vilib>:"Open Config Data.vi"("configuration file path"=w16) -> ("error out"=w20:errorcluster, "refnum"=w17:T8)  [unwired: 8 in, 1 out]
  n163 = vi-ref "斯坦道多参数.lvlib:五参数标样核查.vi"() -> (w12:refnum<vi>)
  n164 = vi-ref "多参数断电保存全局变量.vi"() -> (w18:refnum<vi>)
  n165 = call <userlib>:"Read Panel from INI__ogtk.vi"("error in (no error)"=w20, "VI ref"=w18, "refnum"=w17) -> ("error out"=w21:errorcluster, "refnum out"=w19:T8)  [unwired: 7 in]
  n166 = property on="打开串口" class="Bool (严格)"("Val(Sgnl)"=TRUE ("值(信号)")) -> (error out=w22:errorcluster)  [unwired: 2 in, 1 out]
  n167 = call <vilib>:"Close Config Data.vi"("error in (no error)"=w21, "refnum"=w19) -> ("error out"=w13:errorcluster)  [unwired: 8 in, 1 out]
  n168 = Obtain Notifier(name (unnamed)="MPFlow" ("名称（未命名）"), notification data type=FALSE) -> (notifier out=w25:refnum<notifier>)  [unwired: 2 in, 2 out]
  n169 = control-ref of="控制命令区探头选择"() -> (w24:refnum<vi>)
  n170 = Obtain Queue(name (unnamed)="Mp Task" ("名称（未命名）"), element data type=T2 {"测量模式"=enum."水样测试", "数据类型"="N", "手动启动标记"=FALSE, "测量时间"=3.0} ("启动参数")) -> (queue out=w9:refnum<queue>)  [unwired: 3 in, 2 out]
  n171 = while {
    stop <- FALSE stop-if-true
    n172 = global read "多参数全局变量.vi" "叶绿素数据区"() -> (w355:T7)
    n173 = global read "多参数全局变量.vi" "藻密度数据区"() -> (w354:T7)
    n174 = global read "多参数全局变量.vi" "Cond数据区"() -> (w359:T7)
    n175 = Wait (ms)(milliseconds to wait=u32 5000 ("等待时间（毫秒）")) -> ()  [unwired: 1 out]
    n176 = global read "多参数全局变量.vi" "Turb数据区"() -> (w356:T7)
    n177 = global read "多参数断电保存全局变量.vi" "电导率参数"() -> (w351:T9)
    n178 = global read "多参数断电保存全局变量.vi" "溶解氧参数"() -> (w350:T9)
    n179 = global read "多参数断电保存全局变量.vi" "叶绿素参数"() -> (w347:T9)
    n180 = global read "多参数断电保存全局变量.vi" "藻密度参数"() -> (w346:T9)
    n181 = global read "多参数全局变量.vi" "水温数据区"() -> (w357:T7)
    n182 = global read "多参数全局变量.vi" "ORP数据区"() -> (w353:T7)
    n183 = global read "多参数全局变量.vi" "DO数据区"() -> (w358:T7)
    n184 = global read "多参数全局变量.vi" "pH数据区"() -> (w360:T7)
    n185 = global read "多参数断电保存全局变量.vi" "水温参数"() -> (w349:T9)
    n186 = global read "多参数断电保存全局变量.vi" "浊度参数"() -> (w348:T9)
    n187 = global read "多参数断电保存全局变量.vi" "ORP参数"() -> (w345:T9)
    n188 = global read "多参数断电保存全局变量.vi" "PH参数"() -> (w352:T9)
    n189 = Build Array(w352, w351, w350, w349, w348, w347, w346, w345) -> (w344:T10)
    n190 = Build Array(w360, w359, w358, w357, w356, w355, w354, w353) -> (w343:T11)
    n191 = for {
      tunnel: w344 -> [w365] mode=indexing
      tunnel: w343 -> [w364] mode=indexing
      tunnel: [w363] -> w342 mode=indexing
      n192 = Unbundle By Name(w364) -> ("K"=w369:sgl, "B"=w368:sgl)
      n193 = Bundle By Name(cluster=w365, "曲线截距"=w369, "曲线斜率"=w368, "线性相关系数"=1.0, "二次多项式系数"=0.0) -> (w363:T9)
    }
    n194 = Index Array(array=w342) -> (element #1=w341:T9, element #2=w340:T9, element #3=w339:T9, element #4=w338:T9, element #5=w337:T9, element #6=w336:T9, element #7=w335:T9, element #8=w334:T9)  [unwired: 8 in]
    n195 = global write "多参数断电保存全局变量.vi" "PH参数"(w341) -> ()
    n196 = global write "多参数断电保存全局变量.vi" "电导率参数"(w340) -> ()
    n197 = global write "多参数断电保存全局变量.vi" "溶解氧参数"(w339) -> ()
    n198 = global write "多参数断电保存全局变量.vi" "水温参数"(w338) -> ()
    n199 = global write "多参数断电保存全局变量.vi" "浊度参数"(w337) -> ()
    n200 = global write "多参数断电保存全局变量.vi" "叶绿素参数"(w336) -> ()
    n201 = global write "多参数断电保存全局变量.vi" "藻密度参数"(w335) -> ()
    n202 = global write "多参数断电保存全局变量.vi" "ORP参数"(w334) -> ()
  }
  n203 = while {
    tunnel: w25 -> [w373]
    tunnel: w24 -> [w372]
    tunnel: w22 -> [_]
    tunnel: w13 -> [_]
    tunnel: w12 -> [w371]
    tunnel: w9 -> [w370]
    stop <- FALSE stop-if-true
    n204 = event shown="[6] \"串口设置\": 值改变" {
      selector: _ -> [_ _ _ _ _ _ _ _ _ _ _ _ _ _ _ _ _ _ _ _ _ _ _ _]
      dyn-events: _ -> [_ _ _ _ _ _ _ _ _ _ _ _ _ _ _ _ _ _ _ _ _ _ _ _]
      timeout: _ -> [_ _ _ _ _ _ _ _ _ _ _ _ _ _ _ _ _ _ _ _ _ _ _ _]
      tunnel: w373 -> [_ _ _ _ _ _ _ _ _ _ _ _ _ w525 _ _ _ _ _ _ _ _ _ _]
      tunnel: w372 -> [_ _ w382 w386 _ _ _ _ _ _ _ _ _ _ _ _ _ _ _ _ _ _ w564 w571]
      tunnel: w371 -> [_ _ _ _ _ _ _ _ _ _ _ _ w501 _ _ _ _ _ _ _ _ _ _ _]
      tunnel: w370 -> [_ _ _ _ _ _ _ _ _ _ _ w487 _ _ _ _ _ _ _ _ _ _ _ _]
      event Timeout {
        n205 = event-data() -> ()  [unwired: 1 in, 3 out]
      }
      event "K", "B", "水深校准": Mouse Down {
        n206 = event-data() -> ("CtlRef"=w378:refnum<vi>)  [unwired: 1 in, 7 out]
        n207 = property class="DigNum (严格)"(reference=w378) -> (reference out=w376:refnum<vi>, "Value"=w377:dbl)  [unwired: 1 in, 1 out]
        n208 = call "数字键盘.vi"("OldNumber"=w377) -> ("NewNumber"=w375:dbl)
        n209 = property class="DigNum (严格)"(reference=w376, "Value"=w375) -> ()  [unwired: 1 in, 2 out]
      }
      event "读取": Value Change {
        n210 = event-data() -> ()  [unwired: 1 in, 6 out]
        n211 = property class="Ring (严格)"(reference=w382) -> ("Value"=w381:u16)  [unwired: 1 in, 2 out]
        n212 = call "多参校准读取.vi"("站号"=w381) -> ("B"=w379:dbl, "K"=w380:dbl)  [unwired: 8 in, 1 out]
        n213 = local write "K"(w380) -> ()
        n214 = local write "B"(w379) -> ()
      }
      event "写入": Value Change {
        n215 = event-data() -> ()  [unwired: 1 in, 6 out]
        n216 = property class="Ring (严格)"(reference=w386) -> ("Value"=w385:u16)  [unwired: 1 in, 2 out]
        n217 = call "多参数校准写入.vi"("B"="B", "K"="K", "站号"=w385) -> ()  [unwired: 8 in, 1 out]
      }
      event "水深读取": Value Change {
        w388 = u16 9 items=["氨氮"=3, "水温"=9, "pH值"=10, "溶解氧"=11, "电导率"=12, "浊度"=13, "叶绿素a"=14, "藻密度"=15, "蓝绿藻"=16, "氧化还原电位"=17, "溶解氧%"=18, "盐度"=19] ("站号")
        n218 = event-data() -> ()  [unwired: 1 in, 6 out]
        n219 = call "多参水深校准读取.vi"("站号"=w388) -> ("B"=w387:dbl)  [unwired: 8 in, 2 out]
        n220 = local write "水深校准"(w387) -> ()
      }
      event "水深写入": Value Change {
        w390 = u16 9 items=["氨氮"=3, "水温"=9, "pH值"=10, "溶解氧"=11, "电导率"=12, "浊度"=13, "叶绿素a"=14, "藻密度"=15, "蓝绿藻"=16, "氧化还原电位"=17, "溶解氧%"=18, "盐度"=19] ("站号")
        n221 = event-data() -> ()  [unwired: 1 in, 6 out]
        n222 = call "多参数水深校准写入.vi"("K"="水深校准", "站号"=w390) -> ()  [unwired: 9 in, 1 out]
      }
      event "串口设置": Value Change {
        n223 = event-data() -> ()  [unwired: 1 in, 6 out]
        n224 = global read "多参数断电保存全局变量.vi" "VISA Resource"() -> (w393:refnum<visa-resource-name>)
        n225 = call "串口配置.vi"("VISA资源名称"=w393) -> ("确认 2"=w392:bool, "VISA资源名称 2"=w391:refnum<visa-resource-name>)  [unwired: 9 in]
        n226 = case shown="真" w392 {
          tunnel: w391 -> [_ w394]
          frame False {
          }
          frame True {
            n227 = flat-sequence {
              tunnel: w394 -> [w395]
              frame #0 {
                n228 = global write "多参数断电保存全局变量.vi" "VISA Resource"(w395) -> ()
              }
              frame #1 {
                n229 = call "多参数通讯.vi"("STEP"=enum16{"open", "read", "write", "close"}."open") -> ("error out"=w397:errorcluster)  [unwired: 8 in, 2 out]
                n230 = case shown="错误" w397 {
                  frame No Error {
                  }
                  frame Error {
                    n231 = One Button Dialog(message="多参数串口打开失败" ("消息")) -> ()  [unwired: 1 in, 1 out]
                  }
                }
              }
              frame #2 {
                n232 = call <vilib>:"Application Directory.vi"() -> ("Application Directory"=w412:path)
                n233 = Build Path(base path=w412, name or relative path="data\\sys.ini" ("名称或相对路径")) -> (appended path=w410:path)
                n234 = call <vilib>:"Open Config Data.vi"("configuration file path"=w410) -> ("error out"=w406:errorcluster, "refnum"=w409:T8)  [unwired: 8 in, 1 out]
                n235 = vi-ref "多参数断电保存全局变量.vi"() -> (w408:refnum<vi>)
                n236 = call <userlib>:"Write Panel to INI__ogtk.vi"("error in (no error)"=w406, "VI ref"=w408, "refnum"=w409) -> ("error out"=w405:errorcluster, "refnum out"=w407:T8)  [unwired: 7 in]
                n237 = call <vilib>:"Close Config Data.vi"("error in (no error)"=w405, "refnum"=w407) -> ("error out"=w400:errorcluster, "file path"=w399:path)  [unwired: 8 in]
                n238 = Open/Create/Replace File(file path (use dialog)=w399, error in=w400) -> (refnum out=w403:refnum<file>, error out=w404:errorcluster)  [unwired: 4 in, 1 out]
                n239 = Flush File(refnum=w403, error in=w404) -> (refnum out=w402:refnum<file>, error out=w401:errorcluster)
                n240 = Close File(refnum=w402, error in=w401) -> ()  [unwired: 2 out]
              }
            }
          }
        }
      }
      event "质控参数设置": Value Change {
        n241 = event-data() -> ()  [unwired: 1 in, 6 out]
        n242 = global read "多参数断电保存全局变量.vi" "质控参数设置"() -> (w413:T14)
        n243 = call "多参数质控参数设置.vi"("质控参数设置"=w413) -> ("输出簇"=w414:T15)  [unwired: 10 in]
        n244 = Unbundle By Name(w414) -> ("确定"=w415:bool)
        n245 = case shown="真" w415 {
          tunnel: w414 -> [_ w417]
          tunnel: w413 -> [_ w416]
          frame False {
          }
          frame True {
            n246 = flat-sequence {
              tunnel: w417 -> [w425]
              tunnel: w416 -> [w424]
              frame #0 {
                n247 = Unbundle By Name(w425) -> ("水温标准液标准浓度"=w423:dbl, "酸碱度标准液标准浓度"=w422:dbl, "溶解氧标准液标准浓度"=w421:dbl, "电导率标准液标准浓度"=w420:dbl, "浊度标准液标准浓度"=w419:dbl)
                n248 = Bundle By Name(cluster=w424, "水温标准液标准浓度"=w423, "酸碱度标准液标准浓度"=w422, "溶解氧标准液标准浓度"=w421, "电导率标准液标准浓度"=w420, "浊度标准液标准浓度"=w419) -> (w418:T14)
                n249 = global write "多参数断电保存全局变量.vi" "质控参数设置"(w418) -> ()
              }
              frame #1 {
                n250 = call <vilib>:"Application Directory.vi"() -> ("Application Directory"=w439:path)
                n251 = Build Path(base path=w439, name or relative path="data\\sys.ini" ("名称或相对路径")) -> (appended path=w437:path)
                n252 = call <vilib>:"Open Config Data.vi"("configuration file path"=w437) -> ("error out"=w433:errorcluster, "refnum"=w436:T8)  [unwired: 8 in, 1 out]
                n253 = vi-ref "多参数断电保存全局变量.vi"() -> (w435:refnum<vi>)
                n254 = call <userlib>:"Write Panel to INI__ogtk.vi"("error in (no error)"=w433, "VI ref"=w435, "refnum"=w436) -> ("error out"=w432:errorcluster, "refnum out"=w434:T8)  [unwired: 7 in]
                n255 = call <vilib>:"Close Config Data.vi"("error in (no error)"=w432, "refnum"=w434) -> ("error out"=w427:errorcluster, "file path"=w426:path)  [unwired: 8 in]
                n256 = Open/Create/Replace File(file path (use dialog)=w426, error in=w427) -> (refnum out=w430:refnum<file>, error out=w431:errorcluster)  [unwired: 4 in, 1 out]
                n257 = Flush File(refnum=w430, error in=w431) -> (refnum out=w429:refnum<file>, error out=w428:errorcluster)
                n258 = Close File(refnum=w429, error in=w428) -> ()  [unwired: 2 out]
              }
            }
          }
        }
      }
      event "仪器参数设置": Value Change {
        n259 = event-data() -> ()  [unwired: 1 in, 6 out]
        n260 = global read "多参数断电保存全局变量.vi" "藻密度参数"() -> (w442:T9)
        n261 = global read "多参数断电保存全局变量.vi" "叶绿素参数"() -> (w444:T9)
        n262 = global read "多参数断电保存全局变量.vi" "电导率参数"() -> (w448:T9)
        n263 = global read "多参数断电保存全局变量.vi" "溶解氧参数"() -> (w447:T9)
        n264 = global read "多参数断电保存全局变量.vi" "ORP参数"() -> (w443:T9)
        n265 = global read "多参数断电保存全局变量.vi" "水温参数"() -> (w446:T9)
        n266 = global read "多参数断电保存全局变量.vi" "PH参数"() -> (w449:T9)
        n267 = global read "多参数断电保存全局变量.vi" "浊度参数"() -> (w445:T9)
        n268 = Build Array(w449, w448, w447, w446, w445, w444, w442, w443) -> (w441:T10)
        n269 = call "仪器参数设置.vi"("仪器参数设置输入"=w441) -> ("确定"=w450:bool, "仪器参数设置输出"=w440:T10)  [unwired: 9 in]
        n270 = case shown="真" w450 {
          tunnel: w440 -> [_ w451]
          frame False {
          }
          frame True {
            n271 = flat-sequence {
              tunnel: w451 -> [w460]
              frame #0 {
                n272 = Index Array(array=w460) -> (element #1=w459:T9, element #2=w458:T9, element #3=w457:T9, element #4=w456:T9, element #5=w455:T9, element #6=w452:T9, element #7=w453:T9, element #8=w454:T9)  [unwired: 8 in]
                n273 = global write "多参数断电保存全局变量.vi" "电导率参数"(w458) -> ()
                n274 = global write "多参数断电保存全局变量.vi" "溶解氧参数"(w457) -> ()
                n275 = global write "多参数断电保存全局变量.vi" "水温参数"(w456) -> ()
                n276 = global write "多参数断电保存全局变量.vi" "PH参数"(w459) -> ()
                n277 = global write "多参数断电保存全局变量.vi" "浊度参数"(w455) -> ()
                n278 = global write "多参数断电保存全局变量.vi" "藻密度参数"(w453) -> ()
                n279 = global write "多参数断电保存全局变量.vi" "叶绿素参数"(w452) -> ()
                n280 = global write "多参数断电保存全局变量.vi" "ORP参数"(w454) -> ()
              }
              frame #1 {
                n281 = call <vilib>:"Application Directory.vi"() -> ("Application Directory"=w474:path)
                n282 = Build Path(base path=w474, name or relative path="data\\sys.ini" ("名称或相对路径")) -> (appended path=w472:path)
                n283 = call <vilib>:"Open Config Data.vi"("configuration file path"=w472) -> ("error out"=w468:errorcluster, "refnum"=w471:T8)  [unwired: 8 in, 1 out]
                n284 = vi-ref "多参数断电保存全局变量.vi"() -> (w470:refnum<vi>)
                n285 = call <userlib>:"Write Panel to INI__ogtk.vi"("error in (no error)"=w468, "VI ref"=w470, "refnum"=w471) -> ("error out"=w467:errorcluster, "refnum out"=w469:T8)  [unwired: 7 in]
                n286 = call <vilib>:"Close Config Data.vi"("error in (no error)"=w467, "refnum"=w469) -> ("error out"=w462:errorcluster, "file path"=w461:path)  [unwired: 8 in]
                n287 = Open/Create/Replace File(file path (use dialog)=w461, error in=w462) -> (refnum out=w465:refnum<file>, error out=w466:errorcluster)  [unwired: 4 in, 1 out]
                n288 = Flush File(refnum=w465, error in=w466) -> (refnum out=w464:refnum<file>, error out=w463:errorcluster)
                n289 = Close File(refnum=w464, error in=w463) -> ()  [unwired: 2 out]
              }
            }
          }
        }
      }
      event "释放串口": Value Change {
        n290 = event-data() -> ("NewVal"=w475:bool)  [unwired: 1 in, 5 out]
        n291 = case shown="真" w475 {
          frame False {
          }
          frame True {
            n292 = call "多参数通讯.vi"("STEP"=enum16{"open", "read", "write", "close"}."close") -> ("error out"=w476:errorcluster)  [unwired: 8 in, 2 out]
            n293 = case shown="无错误" w476 {
              frame No Error {
                n294 = property on="打开串口" class="Bool (严格)"("DisabledEnum"=T12."Enabled" ("禁用")) -> ()  [unwired: 2 in, 2 out]
              }
              frame Error {
              }
            }
          }
        }
      }
      event "打开串口": Value Change {
        n295 = event-data() -> ("NewVal"=w479:bool)  [unwired: 1 in, 5 out]
        n296 = case shown="真" w479 {
          frame False {
          }
          frame True {
            n297 = call "多参数通讯.vi"("STEP"=enum16{"open", "read", "write", "close"}."open") -> ("error out"=w480:errorcluster)  [unwired: 8 in, 2 out]
            n298 = case shown="错误" w480 {
              tunnel: [T12."Disabled and Grayed Out" ("禁用") T12."Enabled" ("禁用")] -> w482
              frame No Error {
              }
              frame Error {
                n299 = One Button Dialog(message="多参数串口打开失败" ("消息")) -> ()  [unwired: 1 in, 1 out]
              }
            }
            n300 = property on="打开串口" class="Bool (严格)"("DisabledEnum"=w482, "Value"=FALSE ("打开串口")) -> ()  [unwired: 2 in, 2 out]
          }
        }
      }
      event "水样测试": Value Change {
        n301 = event-data() -> ()  [unwired: 1 in, 6 out]
        n302 = call "多参数启动参数对话框.vi"() -> ("确认"=w489:bool, "测量时间"=w488:dbl)  [unwired: 10 in]
        n303 = case shown="真" w489 {
          tunnel: w488 -> [_ w497]
          tunnel: w487 -> [_ w491]
          frame False {
          }
          frame True {
            n304 = global read "多参数断电保存全局变量.vi" "运行周期"() -> (w493:T16)
            n305 = Unbundle By Name(w493) -> ("运行模式"=w492:enum16{"维护模式", "常规模式", "应急模式", "质控模式"})
            n306 = case shown="\"常规模式\", 默认" w492 {
              tunnel: ["M" ("数据标记表") "N" ("数据标记表")] -> w496
              frame "维护模式" {
              }
              frame "常规模式", Default {
              }
            }
            n307 = Bundle By Name(cluster=T2 {"测量模式"=enum."水样测试", "数据类型"="N", "手动启动标记"=FALSE, "测量时间"=3.0} ("启动参数"), "数据类型"=w496, "测量时间"=w497, "手动启动标记"=TRUE) -> (w490:T2)
            n308 = Enqueue Element(queue=w491, element=w490) -> ()  [unwired: 2 in, 3 out]
          }
        }
      }
      event "标样核查": Value Change {
        n309 = event-data() -> ()  [unwired: 1 in, 6 out]
        n310 = call "多参数标样核查对话框.vi"() -> ("确认"=w502:bool, "输出参数"=w500:T17)  [unwired: 10 in]
        n311 = case shown="真" w502 {
          tunnel: w501 -> [_ w505]
          tunnel: w500 -> [_ w504]
          frame False {
          }
          frame True {
            n312 = property class="VI"(reference=w505) -> ("Name"=w509:string, "Exec.State"=w507:T18)  [unwired: 1 in, 2 out]
            n313 = Open VI Reference(type specifier VI Refnum (for type only)=refnum<vi> refnum, vi path=w509, options=128 ("选项")) -> (vi reference=w508:refnum<vi>)  [unwired: 3 in, 1 out]
            n314 = case shown="\"Idle\"" w507 {
              tunnel: w508 -> [w512 w520]
              tunnel: [w512 w519] -> w506
              tunnel: w504 -> [_ w516]
              frame "Bad", Default {
                n315 = One Button Dialog(message="仪器已经启动，无需重复启动" ("消息")) -> ()  [unwired: 1 in, 1 out]
              }
              frame "Idle" {
                n316 = global read "多参数断电保存全局变量.vi" "运行周期"() -> (w514:T16)
                n317 = Unbundle By Name(w514) -> ("运行模式"=w513:enum16{"维护模式", "常规模式", "应急模式", "质控模式"})
                n318 = case shown="\"常规模式\", 默认" w513 {
                  tunnel: ["M" ("数据标记表") "N" ("数据标记表")] -> w518
                  frame "维护模式" {
                  }
                  frame "常规模式", Default {
                  }
                }
                n319 = Bundle By Name(cluster=T13 {"测量模式"=enum."标样核查", "数据标记表"="N", "输出参数"={"水温"=FALSE, "pH"=FALSE, "DO"=FALSE, "浊度"=FALSE, "电导率"=FALSE, "保存组数"=0.0}} ("启动参数"), "数据标记表"=w518, "输出参数"=w516) -> (w517:T13)
                n320 = call-by-ref "开始异步调用"(reference=w520, "启动参数"=w517) -> (reference out=w519:refnum<vi>)  [unwired: 12 in, 1 out]
              }
            }
            n321 = Close Reference(reference=w506) -> ()  [unwired: 1 in, 1 out]
          }
        }
      }
      event "停止": Value Change {
        n322 = event-data() -> ()  [unwired: 1 in, 6 out]
        n323 = Two Button Dialog(message="请再一次确认是否停止测量" ("消息")) -> (T button?=w523:bool)  [unwired: 2 in]
        n324 = case shown="真" w523 {
          tunnel: w525 -> [_ w528]
          frame False {
          }
          frame True {
            w526 = u16 11 items=["启动测量（全部）"=1, "初始化（清洗）"=10, "停止测量（全部）"=11, "校时"=13, "启动测量（单个传感器）"=19, "停止测量（单个传感器）"=20] ("控制命令")
            w527 = u16 10 items=["氨氮"=3, "水温"=9, "pH值"=10, "溶解氧"=11, "电导率"=12, "浊度"=13, "叶绿素a"=14, "藻密度"=15, "蓝绿藻"=16, "氧化还原电位"=17, "溶解氧%"=18, "盐度"=19] ("站号")
            n325 = Send Notification(notification=TRUE ("通知"), notifier=w528) -> ()  [unwired: 1 in, 2 out]
            n326 = call "多参数控制命令.vi"("控制命令"=w526, "站号"=w527) -> ()  [unwired: 9 in, 1 out]
          }
        }
      }
      event "设置": Value Change {
        n327 = event-data() -> ()  [unwired: 1 in, 6 out]
        n328 = property on="窗格" class="Pane"("Origin"=T3 {"Horizontal"=0, "Vertical"=628} ("原点")) -> ()  [unwired: 2 in, 2 out]
      }
      event "返回": Value Change {
        n329 = event-data() -> ()  [unwired: 1 in, 6 out]
        n330 = property on="窗格" class="Pane"("Origin"=T3 {"Horizontal"=0, "Vertical"=0} ("原点")) -> ()  [unwired: 2 in, 2 out]
      }
      event "传感器参数读取": Value Change {
        n331 = event-data() -> ()  [unwired: 1 in, 6 out]
        n332 = call "多参数传感器参数读取.vi"() -> ("error out"=w533:errorcluster, "添加的数组"=w532:string[][])  [unwired: 9 in, 1 out]
        n333 = call <vilib>:"General Error Handler.vi"("error in (no error)"=w533) -> ()  [unwired: 10 in, 5 out]
        n334 = property on="传感器区" class="MCListbox (严格)"("ItemNames"=w532) -> ()  [unwired: 2 in, 2 out]
      }
      event "关键参数区读取": Value Change {
        n335 = event-data() -> ()  [unwired: 1 in, 6 out]
        n336 = call "多参数关键参数读取.vi"() -> ("error out"=w534:errorcluster, "添加的数组"=w535:string[][])  [unwired: 10 in]
        n337 = call <vilib>:"General Error Handler.vi"("error in (no error)"=w534) -> ()  [unwired: 10 in, 5 out]
        n338 = property on="关键参数区" class="MCListbox (严格)"("ItemNames"=w535) -> ()  [unwired: 2 in, 2 out]
      }
      event "同步时间": Value Change {
        w536 = u16 13 items=["启动测量（全部）"=1, "初始化（清洗）"=10, "停止测量（全部）"=11, "校时"=13, "启动测量（单个传感器）"=19, "停止测量（单个传感器）"=20] ("控制命令")
        w537 = u16 9 items=["氨氮"=3, "水温"=9, "pH值"=10, "溶解氧"=11, "电导率"=12, "浊度"=13, "叶绿素a"=14, "藻密度"=15, "蓝绿藻"=16, "氧化还原电位"=17, "溶解氧%"=18, "盐度"=19] ("站号")
        n339 = event-data() -> ()  [unwired: 1 in, 6 out]
        n340 = call "多参数控制命令.vi"("控制命令"=w536, "站号"=w537) -> ("error out"=w539:errorcluster)  [unwired: 9 in]
        n341 = case shown="错误" w539 {
          tunnel: ["时间同步成功" ("消息") "时间同步失败" ("消息")] -> w538
          frame No Error {
          }
          frame Error {
          }
        }
        n342 = One Button Dialog(message=w538) -> ()  [unwired: 1 in, 1 out]
      }
      event "启动测量(全部)": Value Change {
        w542 = u16 1 items=["启动测量（全部）"=1, "初始化（清洗）"=10, "停止测量（全部）"=11, "校时"=13, "启动测量（单个传感器）"=19, "停止测量（单个传感器）"=20] ("控制命令")
        w543 = u16 9 items=["氨氮"=3, "水温"=9, "pH值"=10, "溶解氧"=11, "电导率"=12, "浊度"=13, "叶绿素a"=14, "藻密度"=15, "蓝绿藻"=16, "氧化还原电位"=17, "溶解氧%"=18, "盐度"=19] ("站号")
        n343 = event-data() -> ()  [unwired: 1 in, 6 out]
        n344 = call "多参数控制命令.vi"("控制命令"=w542, "站号"=w543) -> ("error out"=w545:errorcluster)  [unwired: 9 in]
        n345 = case shown="无错误" w545 {
          tunnel: ["启动成功" ("消息") "启动失败" ("消息")] -> w544
          frame No Error {
          }
          frame Error {
          }
        }
        n346 = One Button Dialog(message=w544) -> ()  [unwired: 1 in, 1 out]
      }
      event "停止测量(全部)": Value Change {
        w550 = u16 11 items=["启动测量（全部）"=1, "初始化（清洗）"=10, "停止测量（全部）"=11, "校时"=13, "启动测量（单个传感器）"=19, "停止测量（单个传感器）"=20] ("控制命令")
        w551 = u16 9 items=["氨氮"=3, "水温"=9, "pH值"=10, "溶解氧"=11, "电导率"=12, "浊度"=13, "叶绿素a"=14, "藻密度"=15, "蓝绿藻"=16, "氧化还原电位"=17, "溶解氧%"=18, "盐度"=19] ("站号")
        n347 = event-data() -> ()  [unwired: 1 in, 6 out]
        n348 = call "多参数控制命令.vi"("控制命令"=w550, "站号"=w551) -> ("error out"=w549:errorcluster)  [unwired: 9 in]
        n349 = case shown="错误" w549 {
          tunnel: ["停止成功" ("消息") "停止失败" ("消息")] -> w548
          frame No Error {
          }
          frame Error {
          }
        }
        n350 = One Button Dialog(message=w548) -> ()  [unwired: 1 in, 1 out]
      }
      event "初始化(清洗)": Value Change {
        w556 = u16 10 items=["启动测量（全部）"=1, "初始化（清洗）"=10, "停止测量（全部）"=11, "校时"=13, "启动测量（单个传感器）"=19, "停止测量（单个传感器）"=20] ("控制命令")
        w557 = u16 9 items=["氨氮"=3, "水温"=9, "pH值"=10, "溶解氧"=11, "电导率"=12, "浊度"=13, "叶绿素a"=14, "藻密度"=15, "蓝绿藻"=16, "氧化还原电位"=17, "溶解氧%"=18, "盐度"=19] ("站号")
        n351 = event-data() -> ()  [unwired: 1 in, 6 out]
        n352 = call "多参数控制命令.vi"("控制命令"=w556, "站号"=w557) -> ("error out"=w554:errorcluster)  [unwired: 9 in]
        n353 = case shown="错误" w554 {
          tunnel: ["初始化成功" ("消息") "初始化失败" ("消息")] -> w555
          frame No Error {
          }
          frame Error {
          }
        }
        n354 = One Button Dialog(message=w555) -> ()  [unwired: 1 in, 1 out]
      }
      event "启动测量(单探)": Value Change {
        w560 = u16 19 items=["启动测量（全部）"=1, "初始化（清洗）"=10, "停止测量（全部）"=11, "校时"=13, "启动测量（单个传感器）"=19, "停止测量（单个传感器）"=20] ("控制命令")
        n355 = event-data() -> ()  [unwired: 1 in, 6 out]
        n356 = property class="Ring (严格)"(reference=w564) -> ("Value"=w563:u16)  [unwired: 1 in, 2 out]
        n357 = call "多参数控制命令.vi"("控制命令"=w560, "站号"=w563) -> ("error out"=w562:errorcluster)  [unwired: 9 in]
        n358 = case shown="无错误" w562 {
          tunnel: ["启动成功" ("消息") "启动失败" ("消息")] -> w561
          frame No Error {
          }
          frame Error {
          }
        }
        n359 = One Button Dialog(message=w561) -> ()  [unwired: 1 in, 1 out]
      }
      event "停止测量(单探)": Value Change {
        w567 = u16 20 items=["启动测量（全部）"=1, "初始化（清洗）"=10, "停止测量（全部）"=11, "校时"=13, "启动测量（单个传感器）"=19, "停止测量（单个传感器）"=20] ("控制命令")
        n360 = event-data() -> ()  [unwired: 1 in, 6 out]
        n361 = property class="Ring (严格)"(reference=w571) -> ("Value"=w570:u16)  [unwired: 1 in, 2 out]
        n362 = call "多参数控制命令.vi"("控制命令"=w567, "站号"=w570) -> ("error out"=w569:errorcluster)  [unwired: 9 in]
        n363 = case shown="错误" w569 {
          tunnel: ["停止成功" ("消息") "停止失败" ("消息")] -> w568
          frame No Error {
          }
          frame Error {
          }
        }
        n364 = One Button Dialog(message=w568) -> ()  [unwired: 1 in, 1 out]
      }
    }
  }
  n365 = while {
    tunnel: w9 -> [w575]
    stop <- FALSE stop-if-true
    n366 = flat-sequence {
      tunnel: w575 -> [w579]
      tunnel: [w577] -> w574
      frame #0 {
        n367 = Dequeue Element(queue=w579) -> (queue out=w577:refnum<queue>, element=w578:T2)  [unwired: 2 in, 2 out]
        n368 = call "五参数水样测试.vi"("启动参数"=w578) -> ()  [unwired: 11 in]
      }
    }
    n369 = Flush Queue(queue=w574) -> ()  [unwired: 1 in, 3 out]
  }
  n370 = control-ref of="本VI"() -> (w8:refnum<vi>)
  n371 = property class="VI"(reference=w8) -> ("Library.Version"=w7:T19)  [unwired: 1 in, 2 out]
  n372 = Unbundle By Name(w7) -> ("Major"=w5:u16, "Minor"=w4:u16, "Fix"=w3:u16, "Build"=w2:u16)
  n373 = Format Into String(format string="模块版本号：%d.%d.%d.%d" ("格式字符串"), w5, w4, w3, w2) -> (resulting string=→"模块版本号":string)  [unwired: 2 in, 1 out]
